vi "can test2.vi"() -> ()   [LabVIEW 2015]
uses:
  <vilib>/myRIO/Common/Instrument Driver Framework/myRIO v1.0/DIO/typedefs/DIO Channels Enum.ctl
  <vilib>/myRIO/Common/Instrument Driver Framework/myRIO v1.0/DIO/typedefs/DIO Channels List.ctl
  <vilib>/myRIO/Common/Instrument Driver Framework/Utilities/typedefs/Generic FPGA Reference.ctl
  <vilib>/myRIO/Common/Instrument Driver Framework/Utilities/typedefs/myRIO v1.0 Reference.ctl
  <vilib>/myRIO/Common/Instrument Driver Framework/Utilities/typedefs/Hardware Version Enum.ctl
  <vilib>/myRIO/Common/Instrument Driver Framework/Utilities/typedefs/myRIO Generic Hardware Reference.ctl
  <vilib>/myRIO/Instrument Drivers/Onboard IO/DIO/typedefs/DIO Reference.ctl
  <vilib>/myRIO/Instrument Drivers/Onboard IO/DIO/DIO.lvlib
  <vilib>/myRIO/Instrument Drivers/Onboard IO/DIO/vis/myRIO DIO Open.xnode
  <vilib>/myRIO/Common/Instrument Driver Framework/myRIO v1.0/DIO/vis/myRIO v1.1 Open DIO.vi
  <vilib>/userdefined/High Color/nirio_resource_hc.ctl
  <vilib>/myRIO/Instrument Drivers/Onboard IO/PWM/PWM.lvlib
  <vilib>/myRIO/Instrument Drivers/Onboard IO/AO/AO.lvlib
  rio_Global.vi
  <vilib>/Analysis/Matrix/NI_Matrix.lvlib
  <vilib>/Analysis/Matrix/Numeric/Conversions/Array To Matrix - RA2.vi
  <vilib>/Analysis/Matrix/Numeric/Multiply/Multiply - RM,RM.vi
  <vilib>/Analysis/Matrix/Numeric/Add/Add - RM,RM.vi
  <vilib>/Analysis/NI_AALBase.lvlib
  <vilib>/Analysis/baseanly.llb/Real Inverse Matrix.vi
  <vilib>/Analysis/Matrix/Numeric/Subtract/Subtract - RM,RM.vi
  <vilib>/Analysis/Matrix/Numeric/Conversions/Array To Matrix - RA.vi
  <vilib>/Analysis/Matrix/Numeric/Conversions/Matrix To Array - RM.vi
  <vilib>/Analysis/Matrix/Numeric/Multiply/Multiply - R,RM.vi
panel:
  out "Ring":u16(ring) items=["P", "R", "N", "D"]
  out "current gear":string(combo)
  in  "gear input":string(combo)
  in  "upper limit":dbl=1.0 format="%#_13g"
  out "XY Graph":cluster{"Y":dbl[], "Y":dbl[]}[](graph)=[{"Y"=[1.82421875, 1.8301353427767753, 1.835194070339203, 1.8394013252854347, 1.8427635002136231, 1.84528698772192, 1.8469781804084777, 1.8478434708714486, 1.8478892517089844, 1.8471219155192375, 1.84554785490036, 1.8431734624505043, 1.8400051307678222, 1.8360492524504661, 1.8313122200965881, 1.8258004263043404, 1.819520263671875, 1.8124781247973443, 1.8046804022789003, 1.796133488714695, 1.7868437767028809, 1.77681765884161, 1.7660615277290344, 1.7545817759633064, 1.742384796142578, 1.7294769808650017, 1.7158647227287291, 1.701554414331913, 1.686552448272705, 1.6708652171492577, 1.654499113559723, 1.637460530102253, 1.619755859375, 1.6013914939761162, 1.5823738265037537, 1.5627092495560646, 1.5424041557312012, 1.5214649376273155, 1.4998979878425598, 1.4777096989750862, 1.4549064636230469, 1.431494674384594, 1.4074807238578795, 1.3828710046410562, 1.3576719093322753, 1.3318898305296898, 1.3055311608314515, 1.2786022928357124, 1.251109619140625, 1.2230595323443412], "Y"=[0.0, 0.5, 1.0, 1.5, 2.0, 2.5, 3.0, 3.5, 4.0, 4.5, 5.0, 5.5, 6.0, 6.5, 7.0, 7.5, 8.0, 8.5, 9.0, 9.5, 10.0, 10.5, 11.0, 11.5, 12.0, 12.5, 13.0, 13.5, 14.0, 14.5, 15.0, 15.5, 16.0, 16.5, 17.0, 17.5, 18.0, 18.5, 19.0, 19.5, 20.0, 20.5, 21.0, 21.5, 22.0, 22.5, 23.0, 23.5, 24.0, 24.5]}, {"Y"=[-1.22265625, -1.2167396572232247, -1.211680929660797, -1.2074736747145653, -1.2041114997863769, -1.20158801227808, -1.1998968195915223, -1.1990315291285514, -1.1989857482910156, -1.1997530844807625, -1.20132714509964, -1.2037015375494957, -1.2068698692321778, -1.2108257475495339, -1.2155627799034119, -1.2210745736956596, -1.227354736328125, -1.2343968752026557, -1.2421945977210997, -1.250741511285305, -1.2600312232971191, -1.27005734115839, -1.2808134722709656, -1.2922932240366936, -1.304490203857422, -1.3173980191349983, -1.3310102772712709, -1.345320585668087, -1.360322551727295, -1.3760097828507423, -1.392375886440277, -1.409414469897747, -1.427119140625, -1.4454835060238838, -1.4645011734962463, -1.4841657504439354, -1.5044708442687988, -1.5254100623726845, -1.5469770121574402, -1.5691653010249138, -1.5919685363769531, -1.615380325615406, -1.6393942761421205, -1.6640039953589438, -1.6892030906677247, -1.7149851694703102, -1.7413438391685485, -1.7682727071642876, -1.795765380859375, -1.8238154676556588, -1.8524165749549866, -1.8815623101592065, -1.911246280670166, -1.9414620938897134, -1.972203357219696, -2.003463678061962, -2.0352366638183597, -2.0675159218907355, -2.1002950596809384, -2.1335676845908162, -2.167327404022217, -2.2015678253769875, -2.2362825560569766, -2.2714652034640315, -2.307109375, -2.3432086780667305, -2.3797567200660703, -2.4167471083998677, -2.4541734504699706, -2.4920293536782263, -2.530308425426483, -2.5690042731165885, -2.6081105041503907, -2.647620725929737, -2.687528545856476, -2.7278275713324547, -2.7685114097595216, -2.809573668539524, -2.8510079550743104, -2.892807876765728, -2.934967041015625, -2.977479055225849, -3.020337526798248, -3.0635360631346704, -3.107068271636963, -3.150927759706974, -3.1951081347465515, -3.2396030041575434, -3.284405975341797, -3.3295106557011604, -3.3749106526374817, -3.4205995735526087, -3.466571025848389, -3.51281861692667, -3.5593359541893004], "Y"=[0.0, 0.5, 1.0, 1.5, 2.0, 2.5, 3.0, 3.5, 4.0, 4.5, 5.0, 5.5, 6.0, 6.5, 7.0, 7.5, 8.0, 8.5, 9.0, 9.5, 10.0, 10.5, 11.0, 11.5, 12.0, 12.5, 13.0, 13.5, 14.0, 14.5, 15.0, 15.5, 16.0, 16.5, 17.0, 17.5, 18.0, 18.5, 19.0, 19.5, 20.0, 20.5, 21.0, 21.5, 22.0, 22.5, 23.0, 23.5, 24.0, 24.5, 25.0, 25.5, 26.0, 26.5, 27.0, 27.5, 28.0, 28.5, 29.0, 29.5, 30.0, 30.5, 31.0, 31.5, 32.0, 32.5, 33.0, 33.5, 34.0, 34.5, 35.0, 35.5, 36.0, 36.5, 37.0, 37.5, 38.0, 38.5, 39.0, 39.5, 40.0, 40.5, 41.0, 41.5, 42.0, 42.5, 43.0, 43.5, 44.0, 44.5, 45.0, 45.5, 46.0, 46.5, 47.0]}, {"Y"=[-0.94, 0.94, 0.94, -0.94, -0.94], "Y"=[-3.2, -3.2, 1.5, 1.5, -3.2]}, {"Y"=[1.984375, 1.978057861328125, 1.9718017578125, 1.965606689453125, 1.95947265625], "Y"=[0.0, 0.5, 1.0, 1.5, 2.0]}, {"Y"=[-5.28125, -5.267578125, -5.25390625, -5.240234375, -5.2265625], "Y"=[0.0, 0.5, 1.0, 1.5, 2.0]}]
  out "Heading":dbl
  out "H_GPS":dbl
  out "pos":dbl[](array[numeric])
  in  "GPS init":bool=TRUE
  out "pos_gps":dbl[](array[numeric]) format="%#_19f"
  out "dt":dbl
  out "Pos_time 10":i32
  out "ecef ref":dbl[](array[numeric])
  out "map":i32=2
  out "vgain":dbl=1.0
  out "vcount":u64=1
  out "hbias":dbl
  out "hcount":u64=1
  out "get heading":bool
  out "get position":bool
  out "heading error":dbl
  out "h_gps":dbl
  out "rt":dbl
  out "pos error":dbl
  out "POS init":bool
  out "Numeric":dbl
  out "cmd steer":dbl=25.77230806 format="%#_12g"
  in  "lane center":dbl=0.05 format="%#_13g"
  in  "Kf":dbl=0.18 format="%#_13g"
  out "Waveform Chart":dynamicdata(graph)
  out "mdps torque volt":dbl
  out "recomammed Speed [km/h]":dbl
  out "lane both":bool
  in  "gain(<1)":dbl=1.0 format="%#_13g"
  in  "rate limit":dbl=0.006 format="%#_13g"
  in  "deadzone":dbl
  in  "visco":dbl
  in  "Kp":dbl=1.2 format="%#_13g"
  out "VS_CAN":dbl
  out "car":refnum<k5>
  in  "forgetting":dbl format="%#_13g"
  out "mdps str_ang":dbl
  out "eye":refnum<k5>
  out "APV":dbl
  out "PWM GAS":dbl=1000.0 min=1000.0 max=2000.0 step=1.0
  out "Auto":bool
  in  "Manual Steering torque":dbl(slide) min=-0.3 max=0.3 step=0.01 scale=-0.3..0.3
  in  "Steering torque input":bool
  out "T init":i32
  out "T out":i32
  in  "manual speed":dbl
  in  "Velocity input":bool
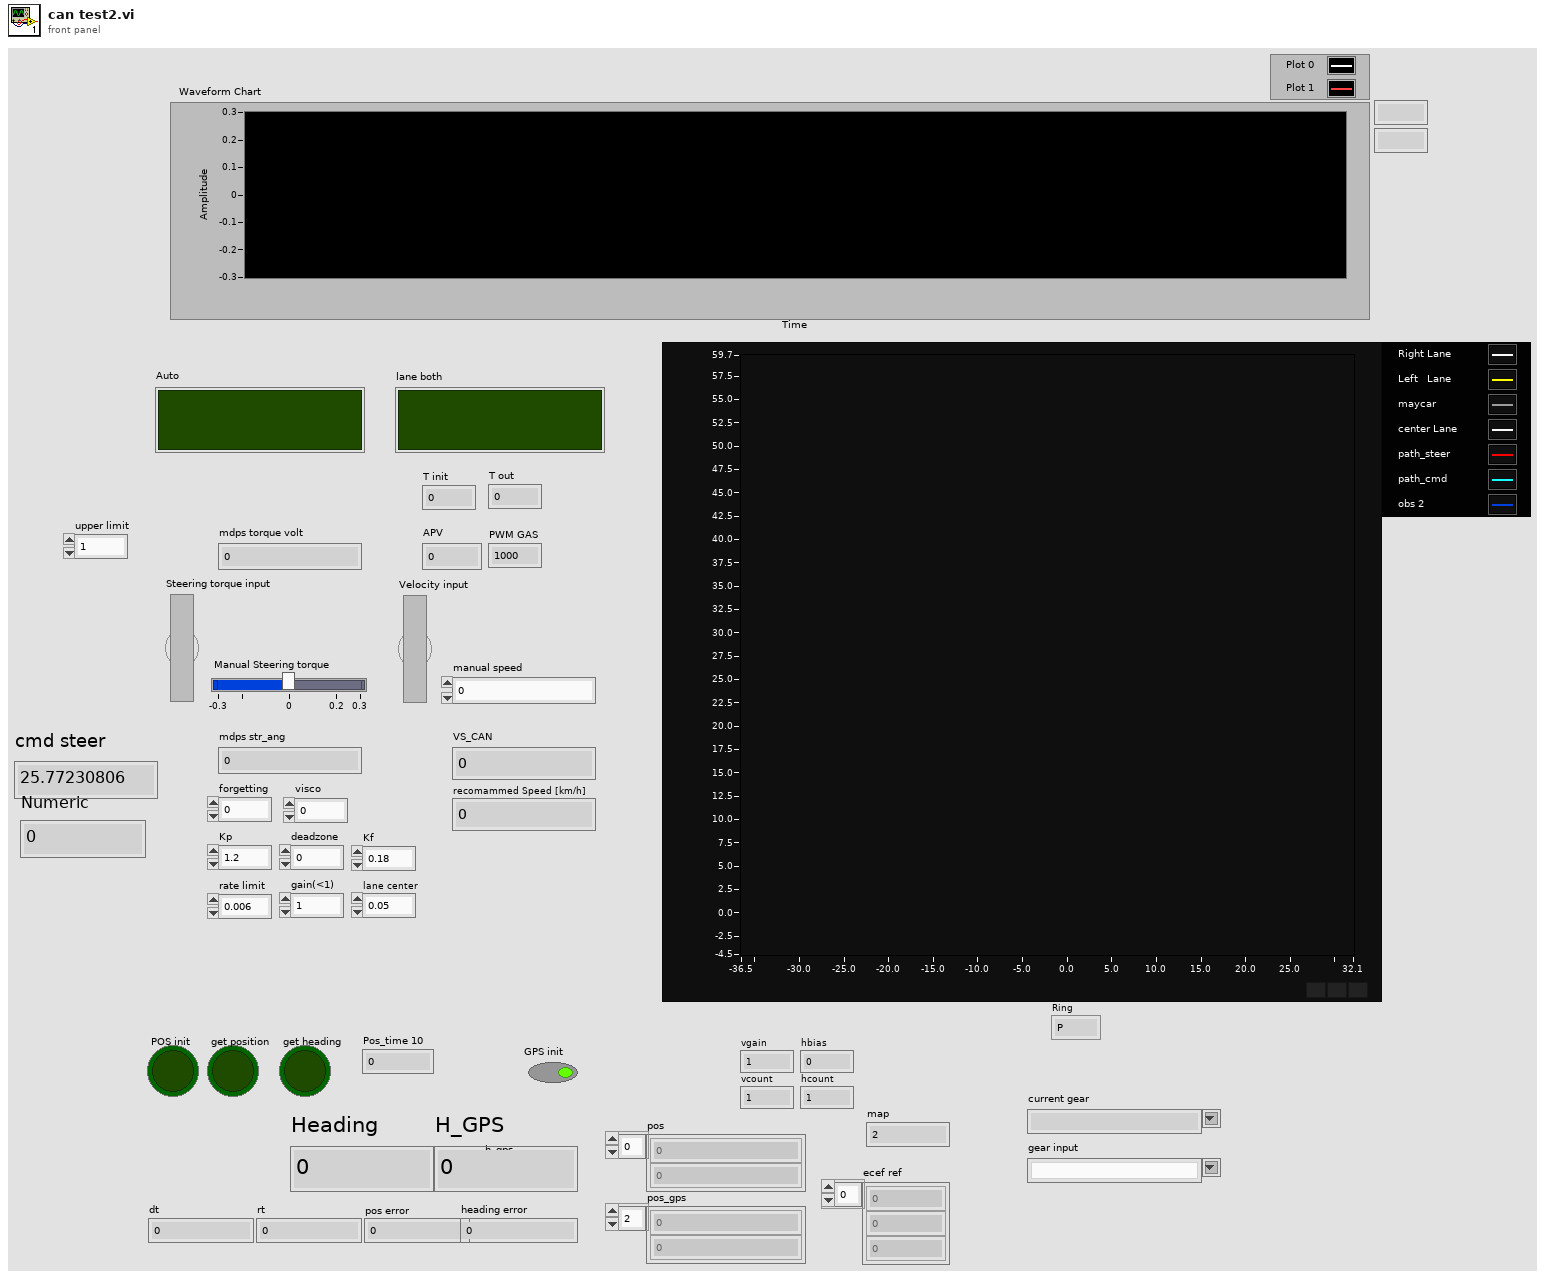
[diagram p1: front panel]
types:
  T1 = enum16{"Standard", "Buffered", "CRLF", "Immediate"}
  T2 = cluster{"identifier":u32, "timestamp":timestamp, "payload":u8[]}
  T3 = typedef "nirio_resource_hc.ctl" = tag
  T4 = typedef "Hardware Version Enum.ctl" = enum16{"Unknown", "myRIO-1900", "myRIO-1950", "roboRIO"}
  T5 = cluster{"connection ID":refnum<k16>, "net address":u32, "port":u16}
  T6 = cluster{"hash":i64, "sys time":i64, "mobileye time":u32, "ID":u32, "data":u8[]}
  T7 = cluster{"hash":i64, "sys time":i64, "car time":u32, "ID":u32, "data":u8[]}
  T8 = typedef "AO.lvlib/AO Reference.ctl" = cluster{"myRIO Reference":T9, "AO Channel List":T12, "AO Scaling Constant List":T14}
  T9 = typedef "myRIO Generic Hardware Reference.ctl" = cluster{"myRIO Model":T4, "myRIO Hardware Reference":T10}
  T10 = typedef "myRIO v1.0 Reference.ctl" = cluster{"Generic FPGA Reference":T11, "Allow multiple opens":bool}
  T11 = typedef "Generic FPGA Reference.ctl" = refnum<k20>
  T12 = typedef "AO Channels List.ctl" = T13[]
  T13 = typedef "AO Channels Enum.ctl" = enum16{"Not Connected", "AudioOut/Left", "AudioOut/Right", "C/AO0", "C/AO1", "A/AO0", "A/AO1", "B/AO0", "B/AO1"}
  T14 = typedef "Analog Scaling Constants List.ctl" = T15[]
  T15 = typedef "Analog Scaling Constants.ctl" = cluster{"LSB Weight (Volts)":dbl, "Offset (Volts)":dbl, "Signed?":bool}
  T16 = typedef "PWM.lvlib/PWM Reference.ctl" = cluster{"myRIO Reference":T9, "PWM Channels Enum":T17, "PWM Configuration":T18}
  T17 = typedef "PWM Channels Enum.ctl" = enum16{"Not Connected", "C/PWM0", "C/PWM1", "A/PWM0", "A/PWM1", "A/PWM2", "B/PWM0", "B/PWM1", "B/PWM2", "PWM/PWM0", "PWM/PWM1", "PWM/PWM2", "PWM/PWM3", "PWM/PWM4", "PWM/PWM5", "PWM/PWM6", "PWM/PWM7", "PWM/PWM8", "PWM/PWM9"}
  T18 = typedef "PWM.lvlib/PWM Configuration.ctl" = cluster{"Frequency":dbl, "Duty Cycle":dbl}
  T19 = typedef "DIO.lvlib/DIO Reference.ctl" = cluster{"myRIO Reference":T9, "DIO Channels List":T20}
  T20 = typedef "DIO Channels List.ctl" = T21[]
  T21 = typedef "DIO Channels Enum.ctl" = enum16{"Not Connected", "C/DIO0", "C/DIO1", "C/DIO2", "C/DIO3", "C/DIO4", "C/DIO5", "C/DIO6", "C/DIO7", "A/DIO0", "A/DIO1", "A/DIO2", "A/DIO3", "A/DIO4", "A/DIO5", "A/DIO6", "A/DIO7", "A/DIO8", "A/DIO9", "A/DIO10", "A/DIO11", "A/DIO12", "A/DIO13", "A/DIO14", "A/DIO15", "B/DIO0", "B/DIO1", "B/DIO2", "B/DIO3", "B/DIO4", "B/DIO5", "B/DIO6", "B/DIO7", "B/DIO8", "B/DIO9", "B/DIO10", "B/DIO11", "B/DIO12", "B/DIO13", "B/DIO14", "B/DIO15", "LED0", "LED1", "LED2", "LED3", "Button0", "DIO/DIO0", "DIO/DIO1", "DIO/DIO2", "DIO/DIO3", "DIO/DIO4", "DIO/DIO5", "DIO/DIO6", "DIO/DIO7", "DIO/DIO8", "DIO/DIO9", "SPI/CS0", "SPI/CS1", "SPI/CS2", "SPI/CS3", "LED RADIO (Green)", "LED RADIO (Red)", "LED COMM (Green)", "LED COMM (Red)", "LED MODE (Green)", "LED MODE (Red)"}
  T22 = cluster{"hash":i64, "sys time":i64, "ref_vel":dbl, "ref_steer":dbl}
  T23 = cluster{"hash":i64, "sys time":i64, "time":dbl, "x":dbl, "y":dbl, "h":dbl, "numSV":i32, "postype":i32, "lag":i32, "hordev":dbl, "lat":dbl, "lon":dbl, "hgt":dbl, "map_idx":i32}
  T24 = cluster{"output[0]":dbl, "output[1]":dbl, "output[2]":dbl, "output[3]":dbl, "output[4]":dbl, "output[5]":dbl, "output[6]":dbl, "output[7]":dbl, "output[8]":dbl, "output[9]":dbl, "output[10]":dbl, "output[11]":dbl, "output[12]":dbl, "output[13]":dbl, "output[14]":dbl}
  T25 = cluster{"hash":i64, "sys time":i64, "time":dbl, "speed":dbl, "heading":dbl, "lat":dbl, "lon":dbl}
  T26 = cluster{"output[0]":dbl, "output[1]":dbl, "output[2]":dbl, "output[3]":dbl, "output[4]":dbl, "output[5]":dbl, "output[6]":dbl}
  T27 = typedef "NI_Matrix.lvlib/RealMatrix.ctl" = dbl[][]
  T28 = cluster{"hash":i64, "sys time":i64, "dt":dbl, "x":dbl, "y":dbl, "speed":dbl, "heading":dbl, "yaw_rate":dbl}
  T29 = cluster{"Real 2D Array[0]":dbl, "Real 2D Array[1]":dbl, "Real 2D Array[2]":dbl, "Real 2D Array[3]":dbl, "Real 2D Array[4]":dbl}
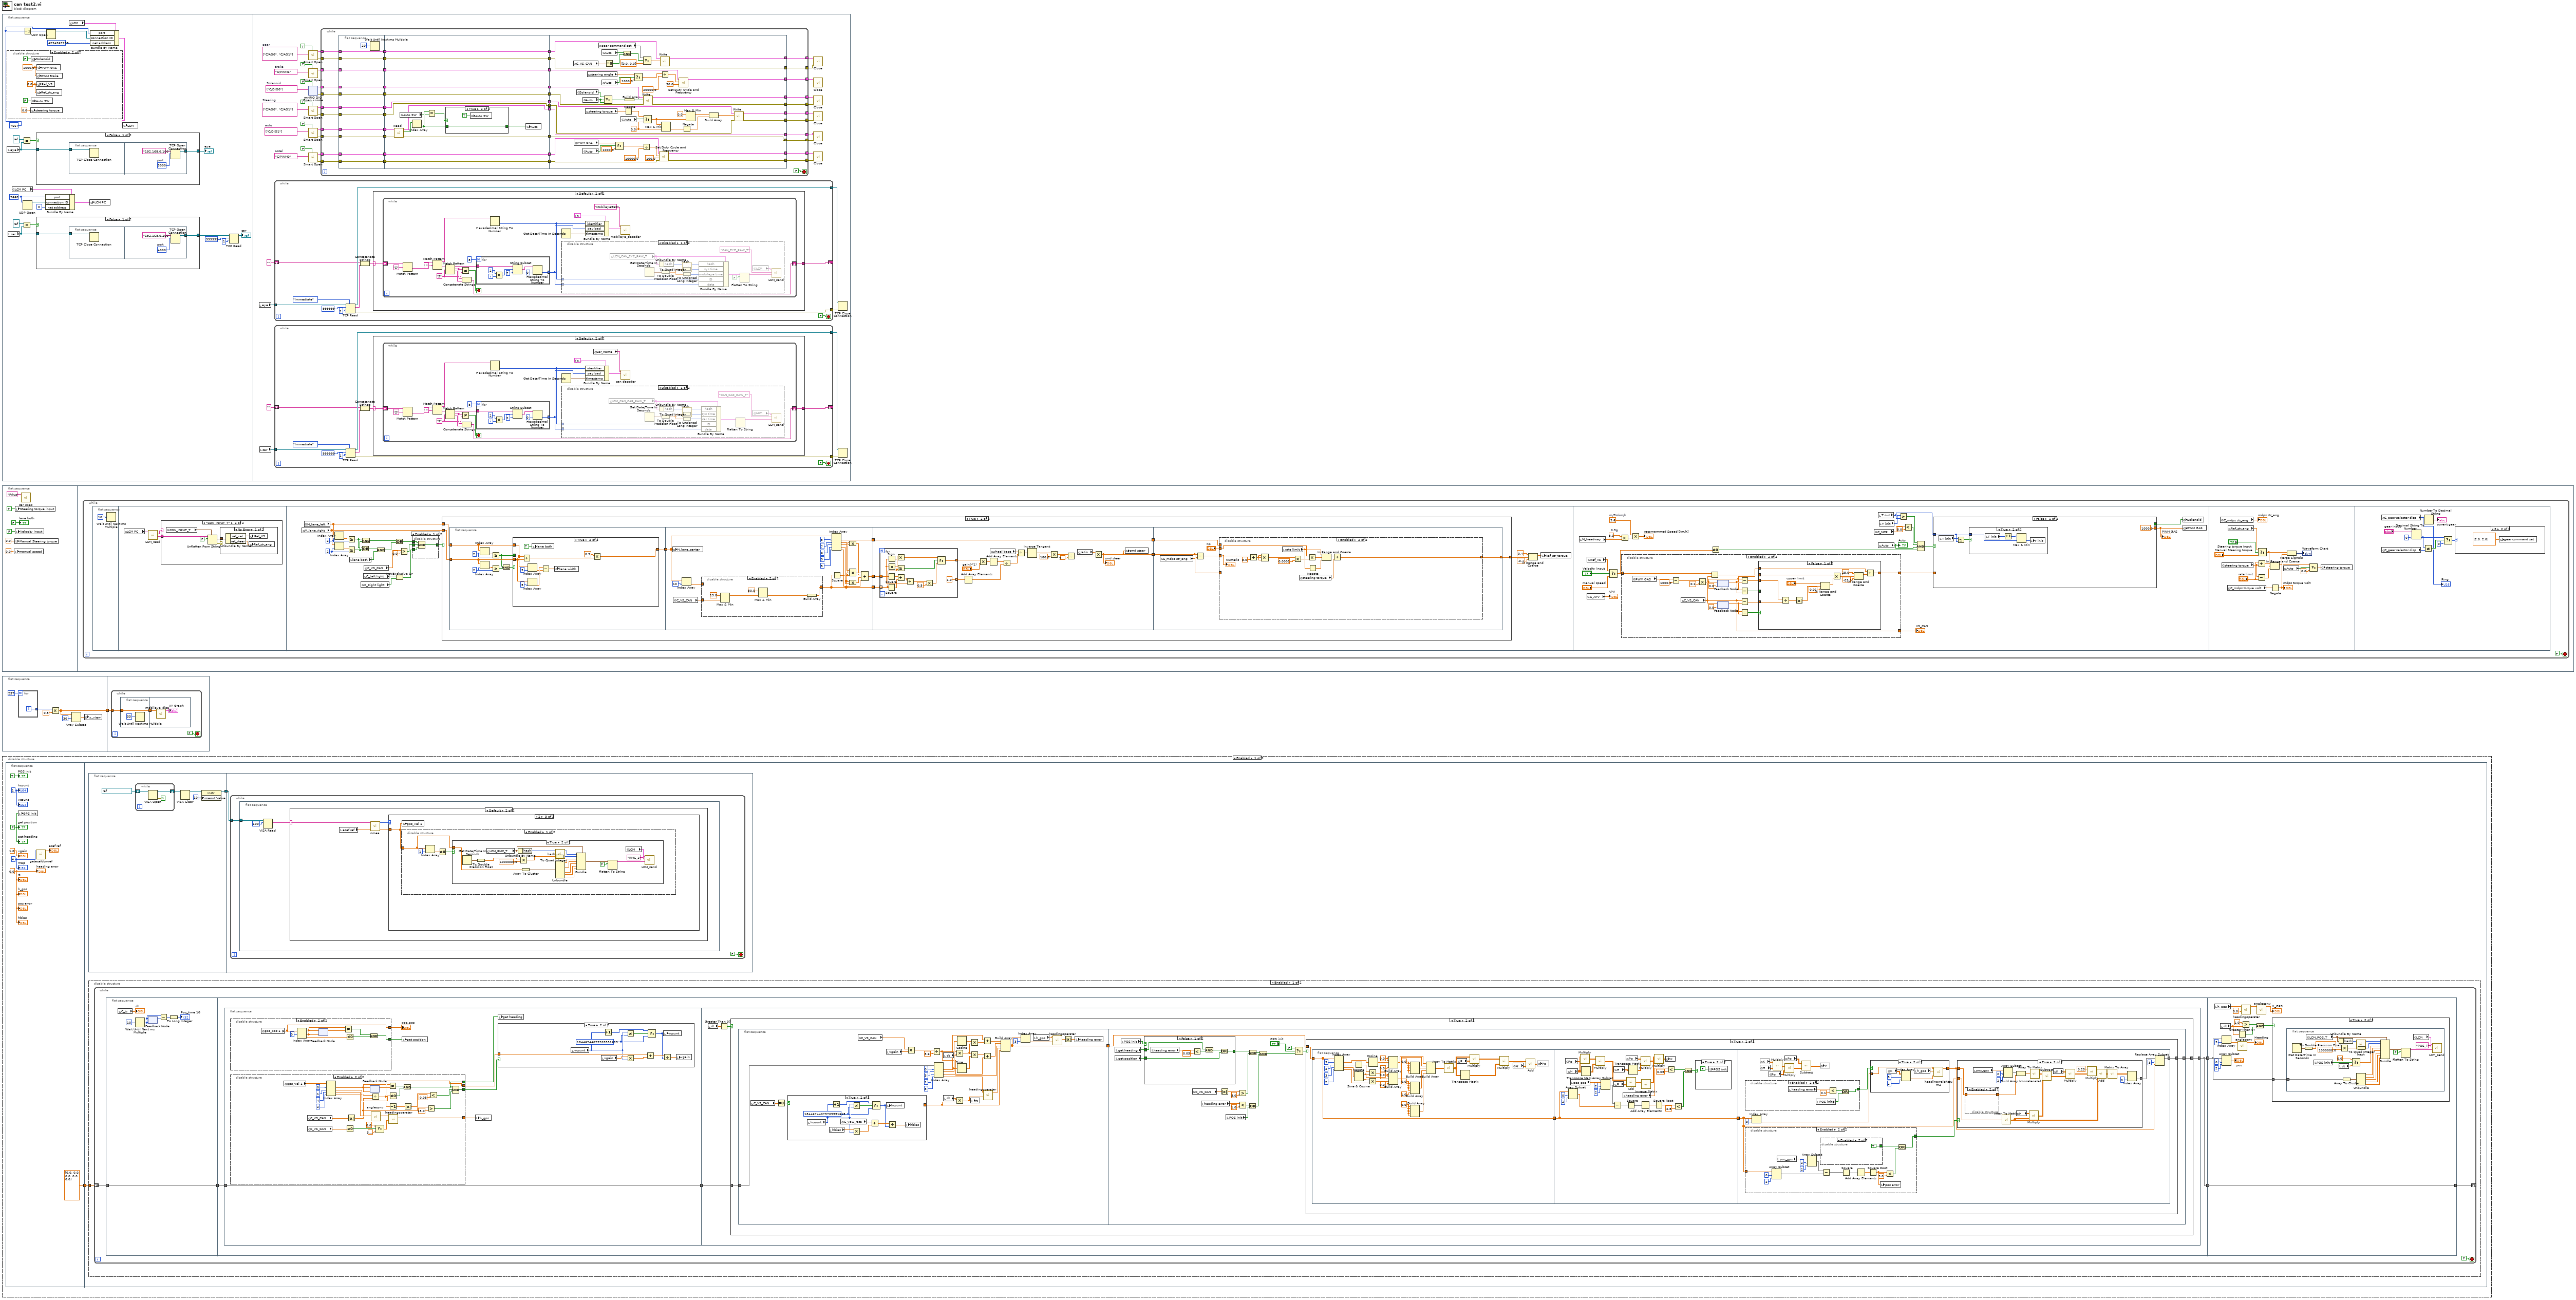
[diagram p0: block diagram]
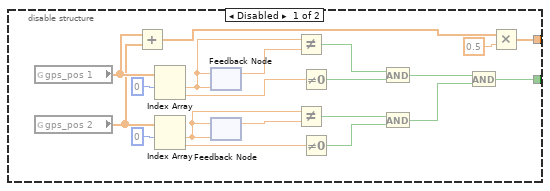
[diagram p2: hidden frame]
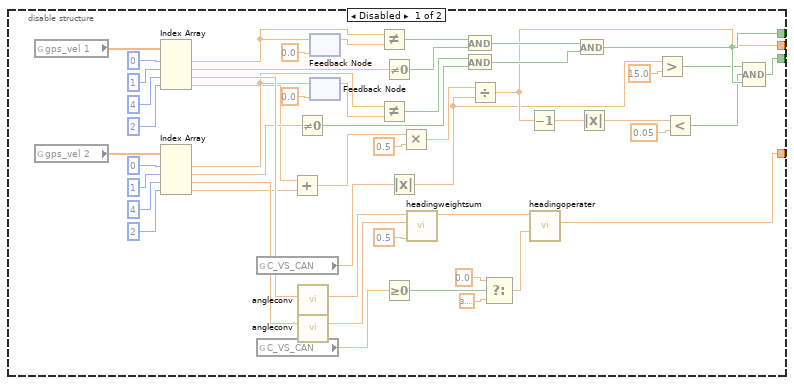
[diagram p3: hidden frame]
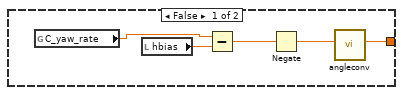
[diagram p6: hidden frame]
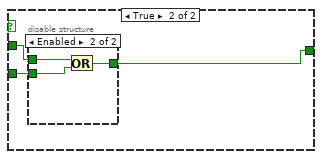
[diagram p7: hidden frame]
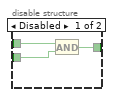
[diagram p8: hidden frame]
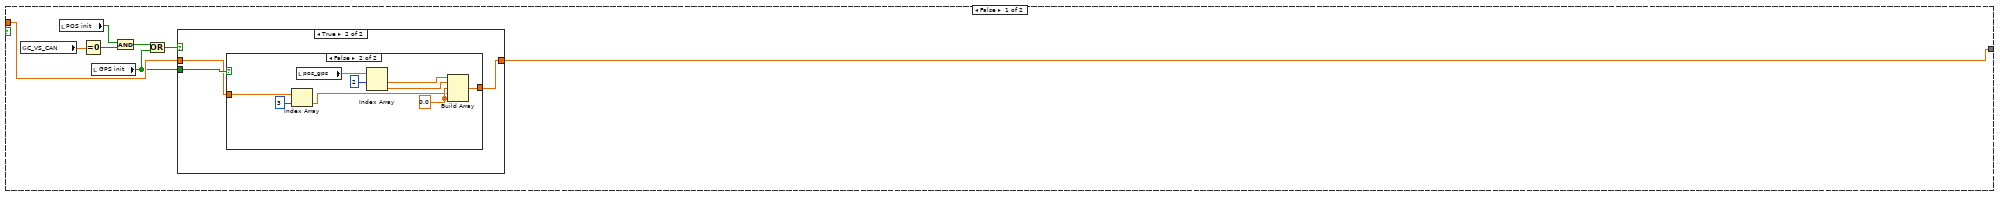
[diagram p9: hidden frame]
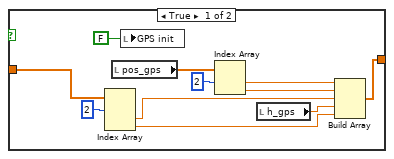
[diagram p11: hidden frame]
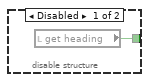
[diagram p13: hidden frame]
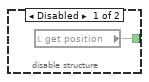
[diagram p14: hidden frame]
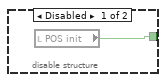
[diagram p15: hidden frame]
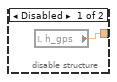
[diagram p17: hidden frame]
diagram:
  n1 = flat-sequence {
    frame #0 {
      w16 = u16 7668 ("port")
      w11 = u16 7667 ("port")
      n2 = disable-structure shown="Enabled" {
        frame Disabled {
        }
        frame Enabled {
          w24 = 0.0 ("Ref_str_ang")
          w25 = 1000.0 ("PWM GAS")
          n3 = global write "rio_Global.vi" "steering torque"(0.0 ("steering")) -> ()
          n4 = global write "rio_Global.vi" "Solenoid"(FALSE ("CAN A 1")) -> ()
          n5 = global write "rio_Global.vi" "Auto SW"(FALSE ("Auto SW")) -> ()
          n6 = global write "rio_Global.vi" "PWM Brake"(w25) -> ()
          n7 = global write "rio_Global.vi" "Ref_str_ang"(w24) -> ()
          n8 = global write "rio_Global.vi" "PWM GAS"(w25) -> ()
          n9 = global write "rio_Global.vi" "Ref_VS"(w24) -> ()
        }
      }
      n10 = local read "eye"() -> (w18:refnum<k5>)
      n11 = local read "car"() -> (w19:refnum<k5>)
      n12 = global read "rio_Global.vi" "LCM PC"() -> (w8:T5)
      n13 = Equal?(x=refnum<k5> refnum ("connection ID"), y=w18) -> (x = y?=w20:bool)
      n14 = Equal?(x=refnum<k5> refnum ("connection ID"), y=w19) -> (x = y?=w22:bool)
      n15 = Decrement(x=w11) -> (x-1=w10:u16)
      n16 = UDP Open(11:w16) -> (port=w14:refnum<k16>)  [unwired: 4 in, 2 out]
      n17 = case shown="False" w20 {
        tunnel: w18 -> [w30 _]
        tunnel: [w29 w35] -> w17
        frame False {
          n18 = flat-sequence {
            tunnel: w30 -> [w31]
            tunnel: [w32] -> w29
            frame #0 {
              n19 = TCP Close Connection(connection ID=w31) -> ()  [unwired: 2 in, 2 out]
            }
            frame #1 {
              w33 = u16 3000  # port
              n20 = TCP Open Connection(address="192.168.0.100", remote port or service name=w33) -> (connection ID=w32:refnum<k5>)  [unwired: 3 in, 1 out]
            }
          }
        }
        frame True {
          w36 = u16 3000  # port
          n21 = TCP Open Connection(address="192.168.0.100", remote port or service name=w36) -> (connection ID=w35:refnum<k5>)  [unwired: 3 in, 1 out]
        }
      }
      "eye" <- w17
      n22 = case shown="False" w22 {
        tunnel: w19 -> [w39 _]
        tunnel: [w38 w44] -> w3
        frame False {
          n23 = flat-sequence {
            tunnel: w39 -> [w40]
            tunnel: [w41] -> w38
            frame #0 {
              n24 = TCP Close Connection(connection ID=w40) -> ()  [unwired: 2 in, 2 out]
            }
            frame #1 {
              w42 = u16 4000  # port
              n25 = TCP Open Connection(address="192.168.0.200", remote port or service name=w42) -> (connection ID=w41:refnum<k5>)  [unwired: 3 in, 1 out]
            }
          }
        }
        frame True {
          w45 = u16 4000  # port
          n26 = TCP Open Connection(address="192.168.0.200", remote port or service name=w45) -> (connection ID=w44:refnum<k5>)  [unwired: 3 in, 1 out]
        }
      }
      n27 = Bundle By Name(cluster=w8, "port"=w16, "connection ID"=w14, "net address"=u32 0) -> (w9:T5)
      n28 = UDP Open(11:w10) -> (port=w13:refnum<k16>)  [unwired: 4 in, 2 out]
      n29 = global read "rio_Global.vi" "LCM"() -> (w7:T5)
      n30 = global write "rio_Global.vi" "LCM PC"(w9) -> ()
      n31 = Bundle By Name(cluster=w7, "port"=w11, "connection ID"=w13, "net address"=u32 4294967295) -> (w6:T5)
      n32 = global write "rio_Global.vi" "LCM"(w6) -> ()
      n33 = TCP Read(connection ID=w3, bytes to read=999999, 9:1 ("timeout ms (25000)")) -> (connection ID out=→"car":refnum<k5>)  [unwired: 2 in, 2 out]
    }
    frame #1 {
      w52 = tag[] ["C/AO0", "C/AO1"]  # gear
      w56 = tag "C/PWM1"  # Brake
      w70 = tag[] ["C/AO0", "C/AO1"]  # Steering
      w77 = tag[] ["C/DIO1"]  # auto
      w82 = tag "C/PWM0"  # Accel
      w87 = tag[] ["C/DIO0"]  # Solenoid
      n34 = local read "eye"() -> (w61:refnum<k5>)
      n35 = local read "car"() -> (w57:refnum<k5>)
      n36 = while {
        tunnel: w61 -> [w146]
        tunnel: [w148] -> w64
        tunnel: [w147] -> w63
        shift-right: [w142] -> _
        shift-left: "" -> [w145]
        stop <- FALSE stop-if-true
        n37 = TCP Read(connection ID=w146, bytes to read=999999, 7:T1."Immediate" ("mode (standard)"), 9:1 ("timeout ms (25000)")) -> (connection ID out=w148:refnum<k5>, data out=w144:string, error out=w147:errorcluster)  [unwired: 1 in]
        n38 = Concatenate Strings(w145, w144) -> (w143:string)
        n39 = case shown="Default" w143 {
          selector: w143 -> [_ w154]
          tunnel: [_ w153] -> w142
          frame "" {
          }
          frame Default {
            n40 = while {
              shift-right: [w161] -> w153
              shift-left: w154 -> [w173]
              stop <- w158 stop-if-true
              w159 = "S" ("regular expression")
              n41 = Match Pattern(string=w173, regular expression="S") -> (after substring=w171:string)  [unwired: 1 in, 3 out]
              n42 = Match Pattern(string=w171, regular expression=" ") -> (before substring=w169:string, after substring=w166:string)  [unwired: 1 in, 2 out]
              n43 = Match Pattern(string=w166, regular expression=w159) -> (before substring=w165:string, match substring=w160:string, after substring=w162:string)  [unwired: 1 in, 1 out]
              n44 = Not Equal?(x=w160, y=w159) -> (x != y?=w158:bool)
              n45 = Concatenate Strings(w160, w162) -> (w161:string)
              n46 = for {
                N: 8 -> [_]
                tunnel: w165 -> [w195]
                tunnel: [w191] -> w155 mode=indexing
                i -> [w190]
                n47 = Multiply(x=2, y=w190) -> (x*y=w193:i32)
                n48 = String Subset(string=w195, offset (0)=w193, length (rest)=2 ("length (rest)")) -> (substring=w188:string)
                n49 = Hexadecimal String To Number(string=w188, default (0uL)=u8 0) -> (number=w191:u8)  [unwired: 1 in, 1 out]
              }
              n50 = Hexadecimal String To Number(string=w169) -> (number=w156:u32)  [unwired: 2 in, 1 out]
              n51 = Get Date/Time In Seconds() -> (seconds since 1Jan1904=w164:timestamp)
              n52 = disable-structure shown="Disabled" {
                disable-tunnel: w156 -> [w175 _]
                disable-tunnel: w155 -> [w174 _]
                frame Disabled {
                  n53 = global read "rio_Global.vi" "LCM_CAN_EYE_RAW_T"() -> (w182:T6)
                  n54 = Get Date/Time In Seconds() -> (seconds since 1Jan1904=w179:timestamp)
                  n55 = Unbundle By Name(w182) -> ("hash"=w181:i64)
                  n56 = To Double Precision Float(number=w179) -> (double precision float=w177:dbl)
                  n57 = To Quad Integer(1:w177) -> (0:w178:i64)
                  n58 = To Unsigned Long Integer(number=w177) -> (unsigned 32bit integer=w176:u32)
                  n59 = call "hash.vi"("input"=w181) -> ("output"=w183:i64)  [unwired: 10 in]
                  n60 = Bundle By Name(cluster=w182, "hash"=w183, "sys time"=w178, "mobileye time"=w176, "ID"=w175, "data"=w174) -> (w185:T6)
                  n61 = Flatten To String(anything=w185, prepend array or string size? (T)=FALSE) -> (data string=w187:string)  [unwired: 2 in, 2 out]
                  n62 = global read "rio_Global.vi" "LCM"() -> (w186:T5)
                  n63 = call "LCM_send.vi"("DATA"=w187, "ID"="CAN_EYE_RAW_T", "LCM"=w186) -> ()  [unwired: 6 in, 3 out]
                }
                frame Enabled {
                }
              }
              n64 = Bundle By Name(cluster=T2 {"identifier"=0, "timestamp"=timestamp(0 s since 1904-01-01), "payload"=[]} ("can cluster"), "identifier"=w156, "payload"=w155, "timestamp"=w164) -> (w163:T2)
              n65 = call "mobileye_decoder.vi"("can cluster"=w163, "name"="Mobileye560") -> ()  [unwired: 10 in]
            }
          }
        }
      }
      n66 = while {
        tunnel: w57 -> [w93]
        tunnel: [w95] -> w58
        tunnel: [w94] -> w59
        shift-right: [w89] -> _
        shift-left: "" -> [w92]
        stop <- FALSE stop-if-true
        n67 = TCP Read(connection ID=w93, bytes to read=999999, 7:T1."Immediate" ("mode (standard)"), 9:1 ("timeout ms (25000)")) -> (connection ID out=w95:refnum<k5>, data out=w91:string, error out=w94:errorcluster)  [unwired: 1 in]
        n68 = Concatenate Strings(w92, w91) -> (w90:string)
        n69 = case shown="Default" w90 {
          selector: w90 -> [_ w101]
          tunnel: [_ w100] -> w89
          frame "" {
          }
          frame Default {
            n70 = while {
              shift-right: [w110] -> w100
              shift-left: w101 -> [w120]
              stop <- w106 stop-if-true
              w107 = "S" ("regular expression")
              n71 = Match Pattern(string=w120, regular expression="S") -> (after substring=w118:string)  [unwired: 1 in, 3 out]
              n72 = Match Pattern(string=w118, regular expression=" ") -> (before substring=w116:string, after substring=w114:string)  [unwired: 1 in, 2 out]
              n73 = Match Pattern(string=w114, regular expression=w107) -> (before substring=w113:string, match substring=w108:string, after substring=w111:string)  [unwired: 1 in, 1 out]
              n74 = Not Equal?(x=w108, y=w107) -> (x != y?=w106:bool)
              n75 = Concatenate Strings(w108, w111) -> (w110:string)
              n76 = for {
                N: 8 -> [_]
                tunnel: w113 -> [w141]
                tunnel: [w137] -> w103 mode=indexing
                i -> [w136]
                n77 = Multiply(x=2, y=w136) -> (x*y=w139:i32)
                n78 = String Subset(string=w141, offset (0)=w139, length (rest)=2 ("length (rest)")) -> (substring=w134:string)
                n79 = Hexadecimal String To Number(string=w134, default (0uL)=u8 0) -> (number=w137:u8)  [unwired: 1 in, 1 out]
              }
              n80 = Hexadecimal String To Number(string=w116) -> (number=w104:u32)  [unwired: 2 in, 1 out]
              n81 = Get Date/Time In Seconds() -> (seconds since 1Jan1904=w112:timestamp)
              n82 = disable-structure shown="Disabled" {
                disable-tunnel: w104 -> [w126 _]
                disable-tunnel: w103 -> [w125 _]
                frame Disabled {
                  n83 = global read "rio_Global.vi" "LCM_CAN_CAR_RAW_T"() -> (w131:T7)
                  n84 = Get Date/Time In Seconds() -> (seconds since 1Jan1904=w133:timestamp)
                  n85 = Unbundle By Name(w131) -> ("hash"=w132:i64)
                  n86 = To Double Precision Float(number=w133) -> (double precision float=w124:dbl)
                  n87 = To Quad Integer(1:w124) -> (0:w128:i64)
                  n88 = To Unsigned Long Integer(number=w124) -> (unsigned 32bit integer=w127:u32)
                  n89 = call "hash.vi"("input"=w132) -> ("output"=w130:i64)  [unwired: 10 in]
                  n90 = Bundle By Name(cluster=w131, "hash"=w130, "sys time"=w128, "car time"=w127, "ID"=w126, "data"=w125) -> (w129:T7)
                  n91 = Flatten To String(anything=w129) -> (data string=w121:string)  [unwired: 3 in, 2 out]
                  n92 = global read "rio_Global.vi" "LCM"() -> (w122:T5)
                  n93 = call "LCM_send.vi"("DATA"=w121, "ID"="CAN_CAR_RAW_T", "LCM"=w122) -> ()  [unwired: 6 in, 3 out]
                }
                frame Enabled {
                }
              }
              n94 = Bundle By Name(cluster=T2 {"identifier"=0, "timestamp"=timestamp(0 s since 1904-01-01), "payload"=[]} ("can cluster"), "identifier"=w104, "payload"=w103, "timestamp"=w112) -> (w109:T2)
              n95 = global read "rio_Global.vi" "Car_name"() -> (w102:string)
              n96 = call "can decoder.vi"("can cluster"=w109, "name"=w102) -> ()  [unwired: 10 in]
            }
          }
        }
      }
      n97 = call <vilib>:"Smart Open.vi"("Allow multiple opens?"=TRUE, "Channel Names"=w52) -> ("error out"=w49:errorcluster, "AO Ref Out"=w50:T8)  [unwired: 8 in]
      n98 = call <vilib>:"Smart Open.vi"("Allow multiple opens?"=FALSE, "Channel Name"=w56) -> ("PWM Ref Out"=w54:T16)  [unwired: 8 in, 1 out]
      n99 = xnode "myRIO DIO Open.xnode"("Allow multiple opens?"=FALSE, "Channel Names"=w87) -> ("error out"=w85:errorcluster, "DIO Ref Out"=w86:T19)  [unwired: 1 in]
      n100 = call <vilib>:"Smart Open.vi"("Allow multiple opens?"=TRUE, "Channel Names"=w70) -> ("error out"=w68:errorcluster, "AO Ref Out"=w69:T8)  [unwired: 8 in]
      n101 = call <vilib>:"Smart Open.vi"("Allow multiple opens?"=FALSE, "Channel Names"=w77) -> ("error out"=w75:errorcluster, "DIO Ref Out"=w76:T19)  [unwired: 8 in]
      n102 = call <vilib>:"Smart Open.vi"("Allow multiple opens?"=FALSE, "Channel Name"=w82) -> ("error out"=w80:errorcluster, "PWM Ref Out"=w81:T16)  [unwired: 8 in]
      n103 = while {
        tunnel: w86 -> [w255]
        tunnel: [w256] -> w84
        tunnel: w85 -> [w254]
        tunnel: [w250] -> w83
        tunnel: w76 -> [w248]
        tunnel: [w246] -> w74
        tunnel: w75 -> [w247]
        tunnel: [w245] -> w73
        tunnel: w69 -> [w244]
        tunnel: [w242] -> w67
        tunnel: w68 -> [w243]
        tunnel: [w241] -> w66
        tunnel: w81 -> [w252]
        tunnel: [w253] -> w79
        tunnel: w80 -> [w251]
        tunnel: [w249] -> w78
        tunnel: w54 -> [w221]
        tunnel: [w220] -> w53
        tunnel: w50 -> [w217]
        tunnel: [w216] -> w48
        tunnel: [w215] -> w47
        tunnel: w49 -> [w212]
        stop <- FALSE ("Auto") stop-if-true
        n104 = flat-sequence {
          tunnel: w243 -> [w261]
          tunnel: w244 -> [w262]
          tunnel: w247 -> [w263]
          tunnel: w248 -> [w264]
          tunnel: w251 -> [w265]
          tunnel: w252 -> [w266]
          tunnel: w254 -> [w267]
          tunnel: w255 -> [w268]
          tunnel: [w268] -> w240
          tunnel: [w267] -> w238
          tunnel: [w266] -> w236
          tunnel: [w265] -> w234
          tunnel: [w264] -> w232
          tunnel: [w263] -> w230
          tunnel: [w262] -> w228
          tunnel: [w261] -> w226
          tunnel: [w259] -> w222
          tunnel: w221 -> [w259]
          tunnel: [w258] -> w218
          tunnel: w217 -> [w258]
          tunnel: [w257] -> w213
          tunnel: w212 -> [w257]
          tunnel: w240 -> [w286]
          tunnel: [w286] -> w239
          tunnel: w238 -> [w285]
          tunnel: [w285] -> w237
          tunnel: w236 -> [w284]
          tunnel: [w284] -> w235
          tunnel: w234 -> [w283]
          tunnel: [w283] -> w233
          tunnel: w232 -> [w279]
          tunnel: [w277] -> w231
          tunnel: w230 -> [w278]
          tunnel: [w276] -> w229
          tunnel: w228 -> [w282]
          tunnel: [w282] -> w227
          tunnel: w226 -> [w281]
          tunnel: [w281] -> w225
          tunnel: [w271] -> w223
          tunnel: w222 -> [w271]
          tunnel: [w270] -> w219
          tunnel: w218 -> [w270]
          tunnel: [w269] -> w214
          tunnel: w213 -> [w269]
          tunnel: [w342] -> w256
          tunnel: [w339] -> w253
          tunnel: [w336] -> w250
          tunnel: [w335] -> w249
          tunnel: [w321] -> w246
          tunnel: [w320] -> w245
          tunnel: [w331] -> w242
          tunnel: [w330] -> w241
          tunnel: w239 -> [w341]
          tunnel: w237 -> [w340]
          tunnel: w235 -> [w338]
          tunnel: w233 -> [w337]
          tunnel: w231 -> [w321]
          tunnel: w229 -> [w320]
          tunnel: w227 -> [w333]
          tunnel: w225 -> [w332]
          tunnel: w223 -> [w306]
          tunnel: [w305] -> w220
          tunnel: w219 -> [w298]
          tunnel: [w297] -> w216
          tunnel: [w296] -> w215
          tunnel: w214 -> [w296]
          frame #0 {
            n105 = Wait Until Next ms Multiple(millisecond multiple=u32 20) -> ()  [unwired: 1 out]
          }
          frame #1 {
            n106 = call <vilib>:"Read.vi"("error in (no error)"=w278, "DIO Ref In"=w279) -> ("error out"=w276:errorcluster, "Values"=w280:bool[], "DIO Ref Out"=w277:T19)  [unwired: 7 in]
            n107 = global read "rio_Global.vi" "Auto SW"() -> (w273:bool)
            n108 = Index Array(array=w280) -> (element=w274:bool)  [unwired: 1 in]
            n109 = Equal?(x=w274, y=w273) -> (x = y?=w275:bool)
            n110 = case shown="True" w275 {
              tunnel: w274 -> [_ w288]
              tunnel: [_ w288] -> w272
              frame False {
              }
              frame True {
                n111 = global write "rio_Global.vi" "Auto SW"(TRUE ("Auto SW")) -> ()
              }
            }
            n112 = global write "rio_Global.vi" "Auto"(w272) -> ()
          }
          frame #2 {
            w318 = 0.0 ("y")
            n113 = global read "rio_Global.vi" "C_VS_CAN"() -> (w292:dbl)
            n114 = global read "rio_Global.vi" "PWM GAS"() -> (w308:dbl)
            n115 = global read "rio_Global.vi" "Solenoid"() -> (w310:bool)
            n116 = global read "rio_Global.vi" "Auto"() -> (w311:bool)
            n117 = global read "rio_Global.vi" "Auto"() -> (w312:bool)
            n118 = global read "rio_Global.vi" "steering torque"() -> (w309:dbl)
            n119 = global read "rio_Global.vi" "steering angle"() -> (w302:dbl)
            n120 = global read "rio_Global.vi" "gear command set"() -> (w295)
            n121 = global read "rio_Global.vi" "Auto"() -> (w290:bool)
            n122 = global read "rio_Global.vi" "Auto"() -> (w300:bool)
            n123 = Select(t=w310, s=w311, f=w311) -> (s? t:f=w314:bool)
            n124 = Equal To 0?(x=w292) -> (x = 0?=w291:bool)
            n125 = Select(t=w308, s=w312, f=1000.0) -> (s? t:f=w317:dbl)
            n126 = global read "rio_Global.vi" "Auto"() -> (w313:bool)
            n127 = And(x=w290, y=w291) -> (x .and. y?=w289:bool)
            n128 = Negate(x=w309) -> (-x=w315:dbl)
            n129 = Build Array(w314) -> (w325:bool[])
            n130 = Select(t=w302, s=w300, f=1000.0) -> (s? t:f=w301:dbl)
            n131 = Divide(x=w317, y=10000.0) -> (x/y=w322:dbl)
            n132 = Select(t=w295, s=w289, f=dbl[] [0.0, 0.0]) -> (s? t:f=w294:dbl[])
            n133 = Select(t=w315, s=w313, f=w318) -> (s? t:f=w319:dbl)
            n134 = call <vilib>:"Write.vi"("error in (no error)"=w340, "Values"=w325, "DIO Ref In"=w341) -> ("error out"=w336:errorcluster, "DIO Ref Out"=w342:T19)  [unwired: 6 in]
            n135 = call <vilib>:"Set Duty Cycle and Frequency.vi"("error in (no error)"=w337, "Frequency [Hz]"=100.0, "Duty Cycle"=w322, "PWM Ref In"=w338) -> ("error out"=w335:errorcluster, "PWM Ref Out"=w339:T16)  [unwired: 5 in]
            n136 = call <vilib>:"Write.vi"("Values"=w294, "AO Ref In"=w298) -> ("AO Ref Out"=w297:T8)  [unwired: 7 in, 1 out]
            n137 = Divide(x=w301, y=20000.0) -> (x/y=w304:dbl)
            n138 = Max & Min(x=w319, y=w318) -> (min(x,y)=w327:dbl)  [unwired: 1 out]
            n139 = call <vilib>:"Set Duty Cycle and Frequency.vi"("Frequency [Hz]"=50.0, "Duty Cycle"=w304, "PWM Ref In"=w306) -> ("PWM Ref Out"=w305:T16)  [unwired: 6 in, 1 out]
            n140 = Negate(x=w327) -> (-x=w326:dbl)
            n141 = Max & Min(x=0.0, y=w319) -> (max(x,y)=w328:dbl)  [unwired: 1 out]
            n142 = Build Array(w328, w326) -> (w334:dbl[])
            n143 = call <vilib>:"Write.vi"("error in (no error)"=w332, "Values"=w334, "AO Ref In"=w333) -> ("error out"=w330:errorcluster, "AO Ref Out"=w331:T8)  [unwired: 6 in]
          }
        }
      }
      n144 = call <vilib>:"Close.vi"("error in (no error)"=w47, "AO Ref In"=w48) -> ()  [unwired: 9 in, 1 out]
      n145 = call <vilib>:"Close.vi"("PWM Ref In"=w53) -> ()  [unwired: 10 in, 1 out]
      n146 = call <vilib>:"Close.vi"("error in (no error)"=w83, "DIO Ref In"=w84) -> ()  [unwired: 9 in, 1 out]
      n147 = call <vilib>:"Close.vi"("error in (no error)"=w66, "AO Ref In"=w67) -> ()  [unwired: 9 in, 1 out]
      n148 = call <vilib>:"Close.vi"("error in (no error)"=w73, "DIO Ref In"=w74) -> ()  [unwired: 9 in, 1 out]
      n149 = call <vilib>:"Close.vi"("error in (no error)"=w78, "PWM Ref In"=w79) -> ()  [unwired: 9 in, 1 out]
      n150 = TCP Close Connection(connection ID=w64, error in (no error)=w63) -> ()  [unwired: 1 in, 2 out]
      n151 = TCP Close Connection(connection ID=w58, error in (no error)=w59) -> ()  [unwired: 1 in, 2 out]
    }
  }
  n152 = flat-sequence {
    frame #0 {
      n153 = local write "manual speed"(0.0 ("manual speed")) -> ()
      n154 = local write "Manual Steering torque"(0.0 ("con_vs")) -> ()
      n155 = local write "Steering torque input"(TRUE ("Steering torque input")) -> ()
      n156 = local write "Velocity input"(FALSE ("Velocity input")) -> ()
      n157 = call "car_spec.vi"("Car_name"="Prius") -> ()  [unwired: 5 in, 6 out]
      "lane both" <- FALSE ("lane both")
    }
    frame #1 {
      n158 = while {
        stop <- FALSE stop-if-true
        n159 = flat-sequence {
          frame #0 {
            n160 = Wait Until Next ms Multiple(millisecond multiple=u32 10) -> ()  [unwired: 1 out]
          }
          frame #1 {
            n161 = global read "rio_Global.vi" "LCM PC"() -> (w353:T5)
            n162 = call "LCM_read.vi"("LCM"=w353) -> ("data"=w351:string, "ID"=w352:string)  [unwired: 7 in, 2 out]
            n163 = case shown="\"CON_INPUT_T\"" w352 {
              tunnel: w351 -> [_ w354]
              frame "False", Default {
              }
              frame "CON_INPUT_T" {
                n164 = global read "rio_Global.vi" "CON_INPUT_T"() -> (w356:T22)
                n165 = Unflatten From String(type=w356, binary string=w354, data includes array or string size? (T)=FALSE) -> (value=w355:T22, error out=w357:errorcluster)  [unwired: 2 in, 1 out]
                n166 = case shown="No Error" w357 {
                  tunnel: w355 -> [w361 _]
                  frame No Error {
                    n167 = Unbundle By Name(w361) -> ("ref_vel"=w360:dbl, "ref_steer"=w359:dbl)
                    n168 = global write "rio_Global.vi" "Ref_str_ang"(w359) -> ()
                    n169 = global write "rio_Global.vi" "Ref_VS"(w360) -> ()
                  }
                  frame Error {
                  }
                }
              }
            }
          }
          frame #2 {
            w382 = 2 ("index")
            w384 = 2 ("index")
            n170 = global read "rio_Global.vi" "M_lane_right"() -> (w367:dbl[])
            n171 = global read "rio_Global.vi" "M_lane_left"() -> (w366:dbl[])
            n172 = Index Array(array=w366, index=w384) -> (element=w385:dbl)
            n173 = Index Array(array=w367, index=w382) -> (element=w383:dbl)
            n174 = Greater Or Equal?(x=w385, y=w384) -> (x >= y?=w373:bool)
            n175 = Greater Or Equal?(x=w383, y=w382) -> (x >= y?=w374:bool)
            n176 = local read "lane both"() -> (w371:bool)
            n177 = Or(x=w373, y=w374) -> (x .or. y?=w372:bool)
            n178 = global read "rio_Global.vi" "C_Right light"() -> (w363:bool)
            n179 = And(x=w373, y=w374) -> (x .and. y?=w370:bool)
            n180 = global read "rio_Global.vi" "C_Left light"() -> (w364:bool)
            n181 = global read "rio_Global.vi" "C_VS_CAN"() -> (w365:dbl)
            n182 = And(x=w372, y=w371) -> (x .and. y?=w369:bool)
            n183 = Or(x=w370, y=w369) -> (x .or. y?=w368:bool)
            n184 = Not Exclusive Or(1:w363, 2:w364) -> (0:w380:bool)
            n185 = Greater?(x=w365, y=0.0) -> (0:w376:bool)
            n186 = disable-structure shown="Enabled" {
              disable-tunnel: [w389 TRUE] -> w381
              disable-tunnel: w380 -> [w388 _]
              disable-tunnel: w376 -> [w387 _]
              disable-tunnel: w368 -> [w386 _]
              frame Enabled {
                n187 = Compound Arithmetic op=AND(w386, w387, w388) -> (w389:bool)
              }
              frame Disabled {
              }
            }
            n188 = case shown="True" w381 {
              tunnel: [w394 w401] -> w377
              tunnel: w366 -> [_ w399]
              tunnel: w367 -> [_ w398]
              frame False {
                n189 = local write "lane both"(FALSE ("lane both")) -> ()
                n190 = global write "rio_Global.vi" "M_lane_center"(dbl[] [] ("M_lane_center")) -> ()
                n191 = global read "rio_Global.vi" "steering torque"() -> (w391:dbl)
                n192 = Multiply(x="forgetting", y=w391) -> (x*y=w394:dbl)
              }
              frame True {
                n193 = flat-sequence {
                  tunnel: [w408] -> w400
                  tunnel: w399 -> [w407]
                  tunnel: w398 -> [w406]
                  tunnel: [w456] -> w404
                  tunnel: [w455] -> w403
                  tunnel: w400 -> [w449]
                  tunnel: [w450] -> w396
                  tunnel: w404 -> [w510]
                  tunnel: w403 -> [w509]
                  tunnel: [w497] -> w402
                  tunnel: [w500] -> w397
                  tunnel: w396 -> [w500]
                  tunnel: w402 -> [w533]
                  tunnel: [w534] -> w401
                  tunnel: w397 -> [w531]
                  frame #0 {
                    w414 = 2 ("index")
                    w412 = 2 ("index")
                    n194 = Index Array(array=w407, index=w412) -> (element=w411:dbl)
                    n195 = Index Array(array=w406, index=w414) -> (element=w413:dbl)
                    n196 = Greater Or Equal?(x=w411, y=w412) -> (x >= y?=w405:bool)
                    n197 = Greater Or Equal?(x=w413, y=w414) -> (x >= y?=w410:bool)
                    n198 = And(x=w405, y=w410) -> (x .and. y?=w409:bool)
                    n199 = case shown="True" w409 {
                      tunnel: w407 -> [w436 w440]
                      tunnel: w406 -> [w431 w444]
                      tunnel: [w428 w445] -> w408
                      tunnel: w405 -> [w430 _]
                      frame False {
                        w423 = 0.2 ("y")
                        w426 = 5 ("index")
                        w435 = 5 ("index")
                        n200 = global read "rio_Global.vi" "overall width"() -> (w415:dbl)
                        n201 = Index Array(array=w436, index=w435) -> (element=w433:dbl)
                        n202 = Index Array(array=w431, index=w426) -> (element=w425:dbl)
                        n203 = global read "rio_Global.vi" "lane width"() -> (w416:dbl)
                        n204 = Multiply(x=w415, y=w423) -> (x*y=w421:dbl)
                        n205 = Add(x=w421, y=w423) -> (x+y=w417:dbl)
                        n206 = Add(x=1.0 ("y"), y=w421) -> (x+y=w418:dbl)
                        n207 = Multiply(x=w416, y=0.5) -> (x*y=w420:dbl)
                        n208 = In Range and Coerce(upper limit=w418, x=w420, lower limit=w417) -> (coerced(x)=w419:dbl)  [unwired: 1 out]
                        n209 = Add(x=w433, y=w419) -> (x+y=w432:dbl)
                        n210 = Subtract(x=w425, y=w419) -> (x-y=w424:dbl)
                        n211 = Replace Array Subset(array=w436, new element=w432, index=w435) -> (w429:dbl[])
                        n212 = Replace Array Subset(array=w431, new element=w424, index=w426) -> (w427:dbl[])
                        n213 = Select(t=w429, s=w430, f=w427) -> (s? t:f=w428:dbl[])
                      }
                      frame True {
                        n214 = Add(x=w440, y=w444) -> (x+y=w447:dbl[])
                        n215 = Index Array(array=w440, index=5) -> (element=w438:dbl)
                        n216 = Index Array(array=w444, index=5) -> (element=w442:dbl)
                        n217 = local write "lane both"(TRUE ("lane both")) -> ()
                        n218 = Subtract(x=w442, y=w438) -> (x-y=w437:dbl)
                        n219 = global write "rio_Global.vi" "lane width"(w437) -> ()
                        n220 = Multiply(x=0.5, y=w447) -> (x*y=w445:dbl[])
                      }
                    }
                  }
                  frame #1 {
                    n221 = global write "rio_Global.vi" "M_lane_center"(w449) -> ()
                    n222 = global read "rio_Global.vi" "C_VS_CAN"() -> (w448:dbl)
                    n223 = Index Array(array=w449, index=10) -> (element=w452:dbl)
                    n224 = disable-structure shown="Enabled" {
                      disable-tunnel: w448 -> [w489 w490]
                      disable-tunnel: [w480 w494] -> w455
                      disable-tunnel: w452 -> [w474 _]
                      frame Disabled {
                        n225 = Subtract(x=w474, y=15.0) -> (x-y=w472:dbl)
                        n226 = Subtract(x=w489, y=15.0) -> (x-y=w483:dbl)
                        n227 = Max & Min(x=w472, y=0.0) -> (max(x,y)=w471:dbl)  [unwired: 1 out]
                        n228 = Max & Min(x=w483, y=0.0) -> (max(x,y)=w482:dbl)  [unwired: 1 out]
                        n229 = Multiply(x=w471, y=2.0) -> (x*y=w479:dbl)
                        n230 = Multiply(x=w482, y=2.0) -> (x*y=w486:dbl)
                        n231 = Round Toward -Infinity(1:w479) -> (0:w470:dbl)
                        n232 = Round Toward -Infinity(1:w486) -> (0:w485:dbl)
                        n233 = Increment(x=w470) -> (x+1=w469:dbl)
                        n234 = Increment(x=w485) -> (x+1=w477:dbl)
                        n235 = global read "rio_Global.vi" "x_view"() -> (w468:dbl[])
                        n236 = Max & Min(x=w469, y=w477) -> (min(x,y)=w476:dbl)  [unwired: 1 out]
                        n237 = Array Subset(array=w468, index=0, length=w476) -> (w480:dbl[])
                      }
                      frame Enabled {
                        n238 = Max & Min(x=15.0, y=w490) -> (max(x,y)=w493:dbl)  [unwired: 1 out]
                        n239 = Max & Min(x=50.0, y=w493) -> (min(x,y)=w492:dbl)  [unwired: 1 out]
                        n240 = Build Array(w492) -> (w494:dbl[])
                      }
                    }
                    n241 = Index Array(array=w449, index #1=5 ("index"), index #2=7 ("index"), index #3=6 ("index"), index #4=9 ("index"), index #5=5 ("index")) -> (element #1=w450:dbl, element #2=w466:dbl, element #3=w464:dbl, element #4=w462:dbl, element #5=w458:dbl)
                    n242 = Square(x=w455) -> (x^2=w454:dbl[])
                    n243 = Compound Arithmetic op=MULTIPLY(w454, w464) -> (w460:dbl[])
                    n244 = Compound Arithmetic op=MULTIPLY(w466, w455, w454) -> (w461:dbl[])
                    n245 = Compound Arithmetic op=MULTIPLY(w455, w462) -> (w459:dbl[])
                    n246 = Compound Arithmetic op=ADD(w461, w460, w459, w458) -> (w456:dbl[])
                  }
                  frame #2 {
                    n247 = for {
                      tunnel: [w516] -> w505 mode=indexing
                      tunnel: w510 -> [w520] mode=indexing
                      tunnel: w509 -> [w518] mode=indexing
                      tunnel: [1.0] -> w504 mode=indexing
                      n248 = Square(x=w520) -> (x^2=w523:dbl)
                      n249 = Square(x=w518) -> (x^2=w524:dbl)
                      n250 = Sign(1:w520) -> (0:w519:dbl)
                      n251 = Absolute Value(x=w520) -> (abs(x)=w522:dbl)
                      n252 = Multiply(x=w518, y=w519) -> (x*y=w517:dbl)
                      n253 = Greater Or Equal?(x=w522, y=w518) -> (x >= y?=w521:bool)
                      n254 = Add(x=w523, y=w524) -> (x+y=w525:dbl)
                      n255 = Divide(x=w525, y=w520) -> (x/y=w526:dbl)
                      n256 = Multiply(x=w526, y=0.5) -> (x*y=w528:dbl)
                      n257 = Select(t=w517, s=w521, f=w528) -> (s? t:f=w516:dbl)
                    }
                    n258 = Add Array Elements(numeric array=w504) -> (sum=w503:dbl)
                    n259 = Multiply(x=w505, y="gain(<1)") -> (x*y=w496:dbl[])
                    n260 = Add Array Elements(numeric array=w496) -> (sum=w507:dbl)
                    n261 = global read "rio_Global.vi" "wheel base"() -> (w499:dbl)
                    n262 = Divide(x=w507, y=w503) -> (x/y=w502:dbl)
                    n263 = Divide(x=w499, y=w502) -> (x/y=w501:dbl)
                    n264 = Inverse Tangent(1:w501) -> (0:w511:dbl)
                    n265 = Multiply(x=w511, y=180.0) -> (x*y=w513:dbl)
                    n266 = Divide(x=w513, y=3.141592653589793) -> (x/y=w508:dbl)
                    n267 = global read "rio_Global.vi" "ratio"() -> (w498:dbl)
                    n268 = Multiply(x=w498, y=w508) -> (x*y=w497:dbl)
                    "cmd steer" <- w497
                    n269 = global write "rio_Global.vi" "cmd steer"(w497) -> ()
                  }
                  frame #3 {
                    n270 = global read "rio_Global.vi" "C_mdps str_ang"() -> (w529:dbl)
                    n271 = Subtract(x=w533, y=w529) -> (x-y=w532:dbl)
                    n272 = disable-structure shown="Enabled" {
                      disable-tunnel: [w547 w585] -> w534
                      disable-tunnel: w533 -> [w545 _]
                      disable-tunnel: w532 -> [w539 w580]
                      disable-tunnel: w531 -> [w537 _]
                      disable-tunnel: "Kp" -> [w535 w586]
                      frame Disabled {
                        n273 = Square(x=w539) -> (x^2=w540:dbl)
                        n274 = Absolute Value(x=w539) -> (abs(x)=w538:dbl)
                        n275 = Multiply(x=w540, y=w539) -> (x*y=w542:dbl)
                        n276 = Greater Or Equal?(x=w538, y=1.0) -> (x >= y?=w543:bool)
                        n277 = Select(t=w542, s=w543, f=w539) -> (s? t:f=w541:dbl)
                        n278 = Multiply(x=w541, y=0.002) -> (x*y=w536:dbl)
                        n279 = Multiply(x=w535, y=w536) -> (x*y=w546:dbl)
                        n280 = disable-structure shown="Disabled" {
                          disable-tunnel: [w555 w574] -> w547
                          disable-tunnel: w546 -> [w549 w575]
                          disable-tunnel: w545 -> [_ w565]
                          disable-tunnel: w537 -> [_ w562]
                          frame Disabled {
                            n281 = Absolute Value(x=w549) -> (abs(x)=w554:dbl)
                            n282 = Greater?(x=w554, y="deadzone") -> (0:w553:bool)
                            n283 = Negate(x="visco") -> (-x=w557:dbl)
                            n284 = Select(t=w549, s=w553, f=0.0) -> (s? t:f=w550:dbl)
                            n285 = call "visco.vi"("min"=w557, "max"="visco", "input"=w550) -> ("output"=w555:dbl)  [unwired: 8 in]
                          }
                          frame Enabled {
                            n286 = Square(x=w565) -> (x^2=w566:dbl)
                            n287 = Multiply(x=w566, y=w565) -> (x*y=w564:dbl)
                            n288 = Multiply(x=w562, y="lane center") -> (x*y=w561:dbl)
                            n289 = Multiply(x=0.002 ("y"), y=w564) -> (x*y=w572:dbl)
                            n290 = In Range and Coerce(upper limit=0.2, x=w561, lower limit=-0.2) -> (coerced(x)=w558:dbl)  [unwired: 1 out]
                            n291 = Multiply(x="Kf", y=w572) -> (x*y=w568:dbl)
                            n292 = In Range and Coerce(upper limit=0.35, x=w568, lower limit=-0.35) -> (coerced(x)=w567:dbl)  [unwired: 1 out]
                            n293 = Compound Arithmetic op=ADD(w558, w567, w575) -> (w574:dbl)
                          }
                        }
                      }
                      frame Enabled {
                        n294 = Divide(x=w580, y=3.0) -> (x/y=w578:dbl)
                        n295 = Compound Arithmetic op=MULTIPLY(w578, w578, w578) -> (w577:dbl)
                        n296 = local read "rate limit"() -> (w583:dbl)
                        n297 = Multiply(x=w577, y=0.0001) -> (x*y=w587:dbl)
                        n298 = global read "rio_Global.vi" "steering torque"() -> (w576:dbl)
                        n299 = Multiply(x=w586, y=w587) -> (x*y=w584:dbl)
                        n300 = Negate(x=w583) -> (-x=w582:dbl)
                        n301 = In Range and Coerce(upper limit=w583, x=w584, lower limit=w582) -> (coerced(x)=w581:dbl)  [unwired: 1 out]
                        n302 = Add(x=w581, y=w576) -> (x+y=w585:dbl)
                        "Numeric" <- w580
                      }
                    }
                  }
                }
              }
            }
            n303 = In Range and Coerce(upper limit=0.4, x=w377, lower limit=-0.4) -> (coerced(x)=w362:dbl)  [unwired: 1 out]
            n304 = global write "rio_Global.vi" "Ref_str_torque"(w362) -> ()
          }
          frame #3 {
            w598 = 3.6  # m/2tokm/h
            w600 = 5.0  # 0.5g
            n305 = global read "rio_Global.vi" "M_headway"() -> (w595:dbl)
            n306 = global read "rio_Global.vi" "C_APV"() -> (→"APV":dbl)
            n307 = global read "rio_Global.vi" "Ref_VS"() -> (w589:dbl)
            n308 = Select(t=w589, s="Velocity input", f="manual speed") -> (s? t:f=w604:dbl)
            n309 = Multiply(x=w600, y=w595) -> (x*y=w599:dbl)
            n310 = disable-structure shown="Enabled" {
              disable-tunnel: w604 -> [w613 w644]
              disable-tunnel: [w612 w641] -> w603
              disable-tunnel: [_ w640] -> w590
              frame Disabled {
                n311 = flat-sequence {
                  tunnel: w613 -> [w638]
                  tunnel: [w637] -> w612
                  frame #0 {
                    w620 = dbl[] [0.016, 0.025, 0.08]  # V_PID_gain
                    n312 = global read "rio_Global.vi" "C_VS_CAN"() -> (w614:dbl)
                    n313 = Subtract(x=w638, y=w614) -> (x-y=w639:dbl)
                    n314 = In Range and Coerce(upper limit=20.0, x=w639, lower limit=-999.0) -> (coerced(x)=w616:dbl)  [unwired: 1 out]
                    n315 = Absolute Value(x=w616) -> (abs(x)=w624:dbl)
                    n316 = feedback #1(w616) -> (w618:dbl)
                    n317 = feedback-in #1(w616) -> ()
                    n318 = Multiply(x=w616, y=0.01) -> (x*y=w634:dbl)
                    n319 = Subtract(x=w616, y=w618) -> (x-y=w617:dbl)
                    n320 = Greater?(x=w624, y=1.0) -> (0:w621:bool)
                    n321 = Select(t=w616, s=w621, f=0.0) -> (s? t:f=w631:dbl)
                    n322 = feedback #2(0.0) -> (w633:dbl)
                    n323 = Multiply(x=w633, y=0.95) -> (x*y=w627:dbl)
                    n324 = Add(x=w627, y=w634) -> (x+y=w628:dbl)
                    n325 = feedback-in #2(w628) -> ()
                    n326 = Divide(x=w617, y=0.01) -> (x/y=w615:dbl)
                    n327 = Build Array(w631, w628, w615) -> (w630:dbl[])
                    n328 = Multiply(x=w620, y=w630) -> (x*y=w629:dbl[])
                    n329 = Add Array Elements(numeric array=w629) -> (sum=w637:dbl)
                  }
                }
              }
              frame Enabled {
                n330 = global read "rio_Global.vi" "PWM GAS"() -> (w656:dbl)
                n331 = Subtract(x=w656, y=1000.0) -> (x-y=w653:dbl)
                n332 = global read "rio_Global.vi" "C_VS_CAN"() -> (w640:dbl)
                n333 = Multiply(x=w653, y=0.1) -> (x*y=w642:dbl)
                n334 = Subtract(x=w644, y=w640) -> (x-y=w643:dbl)
                n335 = feedback-in #3(w642) -> ()
                n336 = feedback #3(0.0) -> (w648:dbl)
                n337 = feedback #4(0.0) -> (w646:dbl)
                n338 = feedback-in #4(w640) -> ()
                n339 = Subtract(x=w642, y=w648) -> (x-y=w647:dbl)
                n340 = Equal?(x=w642, y=w648) -> (x = y?=w649:bool)
                n341 = Subtract(x=w640, y=w646) -> (x-y=w645:dbl)
                n342 = Equal?(x=w640, y=w646) -> (x = y?=w650:bool)
                n343 = case shown="False" w650 {
                  tunnel: w649 -> [_ w674]
                  tunnel: w647 -> [w670 _]
                  tunnel: w645 -> [w669 _]
                  tunnel: w643 -> [w668 w672]
                  tunnel: w642 -> [w667 w671]
                  tunnel: [w666 w673] -> w641
                  frame False {
                    n344 = Divide(x=w670, y=w669) -> (x/y=w661:dbl)
                    n345 = Absolute Value(x=w661) -> (abs(x)=w660:dbl)
                    n346 = In Range and Coerce(upper limit="upper limit", x=w660, lower limit=0.01) -> (coerced(x)=w657:dbl)  [unwired: 1 out]
                    n347 = Multiply(x=w668, y=w657) -> (x*y=w663:dbl)
                    n348 = In Range and Coerce(upper limit=25.0, x=w663, lower limit=-25.0) -> (coerced(x)=w662:dbl)  [unwired: 1 out]
                    n349 = Add(x=w667, y=w662) -> (x+y=w666:dbl)
                  }
                  frame True {
                    n350 = case shown="False" w674 {
                      tunnel: [w679 w684] -> w673
                      tunnel: w672 -> [w678 w683]
                      tunnel: w671 -> [w680 w681]
                      frame False {
                        n351 = In Range and Coerce(upper limit=5.0, x=w678, lower limit=-5.0) -> (coerced(x)=w677:dbl)  [unwired: 1 out]
                        n352 = Add(x=w680, y=w677) -> (x+y=w679:dbl)
                      }
                      frame True {
                        n353 = Equal To 0?(x=w683) -> (x = 0?=w682:bool)
                        n354 = case shown="False" w682 {
                          tunnel: w683 -> [w688 _]
                          tunnel: [w685 w689] -> w684
                          tunnel: w681 -> [_ w689]
                          frame False {
                            n355 = In Range and Coerce(upper limit=1.0, x=w688, lower limit=-1.0) -> (coerced(x)=w685:dbl)  [unwired: 1 out]
                          }
                          frame True {
                          }
                        }
                      }
                    }
                  }
                }
              }
            }
            "VS_CAN" <- w590
            n356 = Multiply(x=w598, y=w599) -> (x*y=→"recomammed Speed [km/h]":dbl)
            n357 = Not Equal To 0?(x=w604) -> (x != 0?=w601:bool)
            n358 = global read "rio_Global.vi" "C_MCP"() -> (w594:dbl)
            n359 = local read "T out"() -> (w606:i32)
            n360 = global read "rio_Global.vi" "Auto"() -> (w593:bool)
            "Auto" <- w593
            n361 = local read "T init"() -> (w605:i32)
            n362 = Greater Or Equal?(x=w605, y=w606) -> (x >= y?=w602:bool)
            n363 = Less?(x=w594, y=5.0) -> (x < y?=w608:bool)
            n364 = Compound Arithmetic op=AND(w602, w608, w593, w601) -> (w607:bool)
            n365 = case shown="False" w607 {
              tunnel: [1000.0 ("Numeric") w703] -> w592
              tunnel: w603 -> [_ w709]
              tunnel: w606 -> [w690 _]
              tunnel: [_ TRUE] -> w591
              frame False {
                n366 = local read "T init"() -> (w691:i32)
                n367 = Less Or Equal?(x=w691, y=w690) -> (x <= y?=w692:bool)
                n368 = case shown="True" w692 {
                  tunnel: w690 -> [_ w695]
                  frame False {
                    n369 = local write "T init"(1 ("T init")) -> ()
                  }
                  frame True {
                    n370 = local read "T init"() -> (w698:i32)
                    n371 = Increment(x=w698) -> (x+1=w697:i32)
                    n372 = Max & Min(x=w697, y=w695) -> (min(x,y)=w696:i32)  [unwired: 1 out]
                    n373 = local write "T init"(w696) -> ()
                  }
                }
              }
              frame True {
                w702 = 1000.0 ("x")
                n374 = disable-structure shown="Enabled" {
                  disable-tunnel: [w715 1000.0 ("PWM GAS")] -> w704
                  frame Disabled {
                    n375 = global read "rio_Global.vi" "PWM GAS"() -> (w715:dbl)
                  }
                  frame Enabled {
                  }
                }
                n376 = Multiply(x=10.0, y=w709) -> (x*y=w707:dbl)
                n377 = Add(x=w707, y=w704) -> (x+y=w706:dbl)
                n378 = In Range and Coerce(upper limit=1700.0, x=w706, lower limit=w702) -> (coerced(x)=w703:dbl)  [unwired: 1 out]
                n379 = Subtract(x=w703, y=w702) -> (x-y=w701:dbl)
                n380 = Multiply(x=w701, y=0.1) -> (x*y=w699:dbl)
                n381 = To Long Integer(number=w699) -> (32bit integer=w711:i32)
                n382 = Add(x=w711, y=20) -> (x+y=w713:i32)
                "T out" <- w713
                n383 = Increment(x=w713) -> (x+1=→"T init":i32)
              }
            }
            "PWM GAS" <- w592
            n384 = global write "rio_Global.vi" "Solenoid"(w591) -> ()
            n385 = global write "rio_Global.vi" "PWM GAS"(w592) -> ()
          }
          frame #4 {
            n386 = global read "rio_Global.vi" "C_mdps str_ang"() -> (→"mdps str_ang":dbl)
            n387 = global read "rio_Global.vi" "steering torque"() -> (w721:dbl)
            n388 = global read "rio_Global.vi" "C_mdps torque volt"() -> (w718:dbl)
            n389 = global read "rio_Global.vi" "Ref_str_ang"() -> (w717:dbl)
            n390 = Add(x="rate limit", y=w721) -> (x+y=w728:dbl)
            n391 = Subtract(x=w721, y="rate limit") -> (x-y=w727:dbl)
            n392 = Select(t=w717, s="Steering torque input", f="Manual Steering torque") -> (s? t:f=w723:dbl)
            n393 = In Range and Coerce(upper limit=w728, x=w723, lower limit=w727) -> (coerced(x)=w724:dbl)  [unwired: 1 out]
            n394 = Negate(x=w718) -> (-x=w726:dbl)
            "mdps torque volt" <- w726
            n395 = global read "rio_Global.vi" "Auto"() -> (w719:bool)
            n396 = Merge Signals(w723, w726) -> (→"Waveform Chart":dynamicdata)
            n397 = Select(t=w724, s=w719, f=0.0) -> (s? t:f=w720:dbl)
            n398 = global write "rio_Global.vi" "steering torque"(w720) -> ()
          }
          frame #5 {
            n399 = global read "rio_Global.vi" "C_gear selector disp"() -> (w733:u8)
            "Ring" <- w733
            n400 = global read "rio_Global.vi" "C_gear selector disp"() -> (w734:u8)
            n401 = Decimal String To Number(string="gear input", default (0L)=u8 0) -> (number=w735:u8)  [unwired: 1 in, 1 out]
            n402 = Not Equal?(x=w735, y=w734) -> (x != y?=w741:bool)
            n403 = Number To Decimal String(number=w733) -> (decimal integer string=→"current gear":string)  [unwired: 1 in]
            n404 = Select(t=w735, s=w741, f=u8 0) -> (s? t:f=w739:u8)
            n405 = case shown="3" w739 {
              frame 1 {
                n406 = global write "rio_Global.vi" "gear command set"(dbl[] [2.0, -2.0]) -> ()
              }
              frame 3 {
                n407 = global write "rio_Global.vi" "gear command set"(dbl[] [2.0, 2.0]) -> ()
              }
              frame 0, Default {
                n408 = global write "rio_Global.vi" "gear command set"(dbl[] [0.0, 0.0] ("gear command set")) -> ()
              }
            }
          }
        }
      }
    }
  }
  n409 = flat-sequence {
    tunnel: [w745] -> w1
    tunnel: w1 -> [w752]
    frame #0 {
      n410 = for {
        N: 257 -> [_]
        tunnel: [w751] -> w749 mode=indexing
        i -> [w751]
      }
      n411 = Multiply(x=w749, y=0.5) -> (x*y=w745:dbl[])
      n412 = Array Subset(array=w745, index=30) -> (w746:dbl[])  [unwired: 1 in]
      n413 = global write "rio_Global.vi" "x_view"(w746) -> ()
    }
    frame #1 {
      n414 = while {
        tunnel: w752 -> [w753]
        stop <- FALSE stop-if-true
        n415 = flat-sequence {
          tunnel: [w756] -> w754
          tunnel: w753 -> [w756]
          tunnel: w754 -> [w758]
          frame #0 {
            n416 = Wait Until Next ms Multiple(millisecond multiple=u32 33) -> ()  [unwired: 1 out]
          }
          frame #1 {
            n417 = call "mobileye_disp.vi"("x_view"=w758) -> ("XY Graph"=→"XY Graph":cluster{"Y":dbl[], "Y":dbl[]}[])  [unwired: 10 in]
          }
        }
      }
    }
  }
  n418 = disable-structure shown="Enabled" {
    frame Enabled {
      n419 = flat-sequence {
        tunnel: [dbl[] [0.0, 0.0, 0.0, 0.0, 0.0] ("pos(i)")] -> w760
        tunnel: w760 -> [w770]
        frame #0 {
          w763 = FALSE ("get heading")
          w764 = u64 1
          w761 = 0.0 ("dh_hat")
          w767 = 4 ("map")
          n420 = local write "GPS init"(w763) -> ()
          n421 = call "getecefdcmref.vi"("map"=w767) -> ("XYZ"=→"ecef ref":dbl[])  [unwired: 10 in, 4 out]
          "map" <- w767
          "vgain" <- 1.0 ("initH")
          "vcount" <- w764
          "hbias" <- w761
          "hcount" <- w764
          "get heading" <- w763
          "get position" <- w763
          "heading error" <- w761
          "h_gps" <- w761
          "rt" <- w761
          "pos error" <- w761
          "POS init" <- TRUE ("POS init")
        }
        frame #1 {
          n422 = flat-sequence {
            tunnel: [w1227] -> w769
            tunnel: w769 -> [w1235]
            frame #0 {
              n423 = while {
                shift-right: [w1233] -> w1229
                shift-left: refnum<visa-resource-name> "ASRL3::INSTR" ("VISA resource name") -> [w1234]
                stop <- w1232 continue-if-true
                n424 = VISA Open(VISA resource name=w1234) -> (VISA resource name=w1233:refnum<visa-resource-name>, error out=w1232:errorcluster)  [unwired: 4 in]
              }
              n425 = VISA Clear(VISA resource name=w1229) -> (VISA resource name out=w1231:refnum<visa-resource-name>)  [unwired: 1 in, 1 out]
              n426 = property class="Instr"(reference=w1231, "General Settings:Timeout Value"=u32 10) -> (reference out=w1227:refnum<visa-resource-name>)  [unwired: 1 in, 1 out]
            }
            frame #1 {
              n427 = while {
                tunnel: w1235 -> [w1236]
                stop <- FALSE stop-if-true
                n428 = flat-sequence {
                  tunnel: w1236 -> [w1238]
                  frame #0 {
                    n429 = VISA Read(VISA resource name=w1238, byte count=u32 100) -> (read buffer=w1239:string)  [unwired: 1 in, 3 out]
                    n430 = case shown="Default" w1239 {
                      selector: w1239 -> [_ w1241]
                      frame "" {
                      }
                      frame Default {
                        n431 = local read "ecef ref"() -> (w1242:dbl[])
                        n432 = call "nmea.vi"("ecef ref"=w1242, "NMEA"=w1241) -> ("output"=w1244:dbl[], "type"=w1243:u32)  [unwired: 8 in]
                        n433 = case shown="2" w1243 {
                          tunnel: w1244 -> [_ w1245 w1280]
                          frame 0, Default {
                          }
                          frame 1 {
                            n434 = disable-structure shown="Enabled" {
                              disable-tunnel: w1245 -> [w1247 _]
                              frame Enabled {
                                n435 = Index Array(array=w1247, index=1) -> (element=w1249:dbl)
                                n436 = Not Equal To 0?(x=w1249) -> (x != 0?=w1246:bool)
                                n437 = case shown="True" w1246 {
                                tunnel: w1247 -> [_ w1269]
                                frame False {
                                }
                                frame True {
                                n438 = Get Date/Time In Seconds() -> (seconds since 1Jan1904=w1254:timestamp)
                                n439 = To Double Precision Float(number=w1254) -> (double precision float=w1253:dbl)
                                n440 = global read "rio_Global.vi" "LCM_GGA_T"() -> (w1278:T23)
                                n441 = Array To Cluster(array=w1269) -> (cluster=w1277:T24)
                                n442 = Unbundle By Name(w1278) -> ("hash"=w1274:i64)
                                n443 = Multiply(x=w1253, y=1000000.0) -> (x*y=w1251:dbl)
                                n444 = Unbundle(w1277) -> ("output[0]"=w1279:dbl, "output[2]"=w1268:dbl, "output[3]"=w1267:dbl, "output[4]"=w1266:dbl, "output[6]"=w1265:dbl, "output[7]"=w1263:dbl, "output[8]"=w1261:dbl, "output[9]"=w1259:dbl, "output[12]"=w1258:dbl, "output[13]"=w1257:dbl, "output[14]"=w1256:dbl)  [unwired: 4 out]
                                n445 = To Quad Integer(1:w1251) -> (0:w1250:i64)
                                n446 = To Long Integer(number=w1265) -> (32bit integer=w1264:i32)
                                n447 = To Long Integer(number=w1263) -> (32bit integer=w1262:i32)
                                n448 = To Long Integer(number=w1261) -> (32bit integer=w1260:i32)
                                n449 = call "hash.vi"("input"=w1274) -> ("output"=w1273:i64)  [unwired: 10 in]
                                n450 = local read "map"() -> (w1255:i32)
                                n451 = Bundle(cluster=w1278, "hash"=w1273, "sys time"=w1250, "time"=w1279, "x"=w1268, "y"=w1267, "h"=w1266, "numSV"=w1264, "postype"=w1262, "lag"=w1260, "hordev"=w1259, "lat"=w1258, "lon"=w1257, "hgt"=w1256, "map_idx"=w1255) -> (w1275:T23)
                                n452 = Flatten To String(anything=w1275, prepend array or string size? (T)=FALSE) -> (data string=w1271:string)  [unwired: 2 in, 2 out]
                                n453 = global read "rio_Global.vi" "LCM"() -> (w1270:T5)
                                n454 = call "LCM_send.vi"("DATA"=w1271, "ID"="GGA_1", "LCM"=w1270) -> ()  [unwired: 6 in, 3 out]
                                }
                                }
                              }
                              frame Disabled {
                              }
                            }
                            n455 = global write "rio_Global.vi" "gps_pos 1"(w1245) -> ()
                          }
                          frame 2 {
                            n456 = disable-structure shown="Enabled" {
                              disable-tunnel: w1280 -> [w1284 _]
                              frame Enabled {
                                n457 = Index Array(array=w1284, index=1) -> (element=w1283:dbl)
                                n458 = Not Equal To 0?(x=w1283) -> (x != 0?=w1281:bool)
                                n459 = case shown="True" w1281 {
                                tunnel: w1284 -> [_ w1303]
                                frame False {
                                }
                                frame True {
                                n460 = Get Date/Time In Seconds() -> (seconds since 1Jan1904=w1289:timestamp)
                                n461 = To Double Precision Float(number=w1289) -> (double precision float=w1288:dbl)
                                n462 = global read "rio_Global.vi" "LCM_RMC_T"() -> (w1304:T25)
                                n463 = Unbundle By Name(w1304) -> ("hash"=w1300:i64)
                                n464 = Multiply(x=w1288, y=1000000.0) -> (x*y=w1286:dbl)
                                n465 = Array To Cluster(array=w1303) -> (cluster=w1302:T26)
                                n466 = To Quad Integer(1:w1286) -> (0:w1285:i64)
                                n467 = call "hash.vi"("input"=w1300) -> ("output"=w1299:i64)  [unwired: 10 in]
                                n468 = Unbundle(w1302) -> ("output[0]"=w1294:dbl, "output[2]"=w1293:dbl, "output[4]"=w1292:dbl, "output[5]"=w1291:dbl, "output[6]"=w1290:dbl)  [unwired: 2 out]
                                n469 = Bundle(cluster=w1304, "hash"=w1299, "sys time"=w1285, "time"=w1294, "speed"=w1293, "heading"=w1292, "lat"=w1291, "lon"=w1290) -> (w1295:T25)
                                n470 = Flatten To String(anything=w1295, prepend array or string size? (T)=FALSE) -> (data string=w1297:string)  [unwired: 2 in, 2 out]
                                n471 = global read "rio_Global.vi" "LCM"() -> (w1296:T5)
                                n472 = call "LCM_send.vi"("DATA"=w1297, "ID"="RMC_1", "LCM"=w1296) -> ()  [unwired: 6 in, 3 out]
                                }
                                }
                              }
                              frame Disabled {
                              }
                            }
                            n473 = global write "rio_Global.vi" "gps_vel 1"(w1280) -> ()
                          }
                        }
                      }
                    }
                  }
                }
              }
            }
          }
          n474 = disable-structure shown="Enabled" {
            disable-tunnel: w770 -> [w771 _]
            frame Enabled {
              n475 = while {
                shift-right: [w772] -> _
                shift-left: w771 -> [w773]
                stop <- FALSE stop-if-true
                n476 = flat-sequence {
                  tunnel: [w784] -> w776
                  tunnel: w773 -> [w784]
                  tunnel: w776 -> [w787]
                  tunnel: [w786] -> w775
                  tunnel: [w786] -> w774
                  tunnel: [w1200] -> w772
                  tunnel: w775 -> [w1201]
                  tunnel: w774 -> [w1200]
                  frame #0 {
                    n477 = global read "rio_Global.vi" "C_ts"() -> (→"dt":dbl)
                    n478 = Wait Until Next ms Multiple(millisecond multiple=u32 10) -> (millisecond timer value=w782:u32)
                    n479 = feedback #5(w782) -> (w781:u32)
                    n480 = feedback-in #5(w782) -> ()
                    n481 = Subtract(x=w782, y=w781) -> (x-y=w780:u32)
                    n482 = To Long Integer(number=w780) -> (32bit integer=→"Pos_time 10":i32)
                  }
                  frame #1 {
                    n483 = flat-sequence {
                      tunnel: w787 -> [w794]
                      tunnel: [w794] -> w785
                      tunnel: [w917] -> w786
                      tunnel: w785 -> [w918]
                      frame #0 {
                        n484 = disable-structure shown="Enabled" {
                          disable-tunnel: [w814 w815] -> w789
                          disable-tunnel: [w795 w816] -> w788
                          frame Disabled {
                            n485 = global read "rio_Global.vi" "gps_pos 1"() -> (w811:dbl[])
                            n486 = global read "rio_Global.vi" "gps_pos 2"() -> (w798:dbl[])
                            n487 = Add(x=w811, y=w798) -> (x+y=w813:dbl[])
                            n488 = Index Array(array=w811, index #1=0 ("index")) -> (element #1=w810:dbl, element #2=w809:dbl)  [unwired: 1 in]
                            n489 = Index Array(array=w798, index #1=0 ("index")) -> (element #1=w799:dbl, element #2=w800:dbl)  [unwired: 1 in]
                            n490 = feedback #6(w810) -> (w808:dbl)
                            n491 = feedback-in #6(w810) -> ()
                            n492 = feedback #7(w799) -> (w801:dbl)
                            n493 = feedback-in #7(w799) -> ()
                            n494 = Not Equal?(x=w810, y=w808) -> (x != y?=w807:bool)
                            n495 = Not Equal?(x=w799, y=w801) -> (x != y?=w802:bool)
                            n496 = Not Equal To 0?(x=w809) -> (x != 0?=w806:bool)
                            n497 = Not Equal To 0?(x=w800) -> (x != 0?=w803:bool)
                            n498 = And(x=w807, y=w806) -> (x .and. y?=w796:bool)
                            n499 = And(x=w802, y=w803) -> (x .and. y?=w797:bool)
                            n500 = And(x=w796, y=w797) -> (x .and. y?=w814:bool)
                            n501 = Multiply(x=w813, y=0.5) -> (x*y=w795:dbl[])
                          }
                          frame Enabled {
                            n502 = global read "rio_Global.vi" "gps_pos 1"() -> (w816:dbl[])
                            n503 = Index Array(array=w816, index #1=0 ("index")) -> (element #1=w822:dbl, element #2=w821:dbl)  [unwired: 1 in]
                            n504 = feedback #8(w822) -> (w820:dbl)
                            n505 = feedback-in #8(w822) -> ()
                            n506 = Not Equal?(x=w822, y=w820) -> (x != y?=w819:bool)
                            n507 = Not Equal To 0?(x=w821) -> (x != 0?=w818:bool)
                            n508 = And(x=w819, y=w818) -> (x .and. y?=w815:bool)
                          }
                        }
                        "pos_gps" <- w788
                        n509 = disable-structure shown="Enabled" {
                          disable-tunnel: [w868 w899] -> w793
                          disable-tunnel: [w867 w878] -> w792
                          disable-tunnel: [w839 w889] -> w791
                          disable-tunnel: [w827 w884] -> w790
                          frame Disabled {
                            n510 = global read "rio_Global.vi" "gps_vel 1"() -> (w866:dbl[])
                            n511 = global read "rio_Global.vi" "gps_vel 2"() -> (w845:dbl[])
                            n512 = Index Array(array=w866, index #1=0 ("index"), index #2=1 ("index"), index #3=4 ("index"), index #4=2 ("index")) -> (element #1=w857:dbl, element #2=w862:dbl, element #3=w859:dbl, element #4=w831:dbl)
                            n513 = Index Array(array=w845, index #1=0 ("index"), index #2=1 ("index"), index #3=4 ("index"), index #4=2 ("index")) -> (element #1=w854:dbl, element #2=w849:dbl, element #3=w852:dbl, element #4=w830:dbl)
                            n514 = global read "rio_Global.vi" "C_VS_CAN"() -> (w824:dbl)
                            n515 = global read "rio_Global.vi" "C_VS_CAN"() -> (w871:dbl)
                            n516 = Add(x=w831, y=w830) -> (x+y=w829:dbl)
                            n517 = Not Equal To 0?(x=w849) -> (x != 0?=w850:bool)
                            n518 = call "angleconv.vi"("deg"=w859) -> ("rad"=w842:dbl)  [unwired: 9 in, 1 out]
                            n519 = call "angleconv.vi"("deg"=w852) -> ("rad"=w841:dbl)  [unwired: 9 in, 1 out]
                            n520 = feedback #9(0.0 ("Real Matrix Element")) -> (w856:dbl)
                            n521 = feedback-in #9(w857) -> ()
                            n522 = feedback #10(0.0 ("Real Matrix Element")) -> (w855:dbl)
                            n523 = feedback-in #10(w854) -> ()
                            n524 = Not Equal?(x=w857, y=w856) -> (x != y?=w863:bool)
                            n525 = Not Equal?(x=w854, y=w855) -> (x != y?=w848:bool)
                            n526 = Not Equal To 0?(x=w862) -> (x != 0?=w861:bool)
                            n527 = Greater Or Equal To 0?(x=w871) -> (x >= 0?=w872:bool)
                            n528 = Absolute Value(x=w824) -> (abs(x)=w823:dbl)
                            n529 = Multiply(x=w829, y=0.5) -> (x*y=w838:dbl)
                            n530 = call "headingweightsum.vi"("a"=0.5, "h1"=w841, "h2"=w842) -> ("a*h2+(1-a)*h1"=w870:dbl)  [unwired: 8 in]
                            n531 = And(x=w863, y=w861) -> (x .and. y?=w844:bool)
                            n532 = And(x=w848, y=w850) -> (x .and. y?=w843:bool)
                            n533 = Divide(x=w838, y=w823) -> (x/y=w839:dbl)
                            n534 = Select(t=0.0, s=w872, f=3.141592653589793) -> (s? t:f=w869:dbl)
                            n535 = Decrement(x=w839) -> (x-1=w835:dbl)
                            n536 = call "headingoperater.vi"("h1"=w869, "h2"=w870) -> ("h2-h1"=w868:dbl)  [unwired: 8 in, 1 out]
                            n537 = And(x=w844, y=w843) -> (x .and. y?=w867:bool)
                            n538 = Absolute Value(x=w835) -> (abs(x)=w836:dbl)
                            n539 = Greater?(x=w823, y=15.0) -> (0:w825:bool)
                            n540 = Less?(x=w836, y=0.05) -> (x < y?=w828:bool)
                            n541 = Compound Arithmetic op=AND(w825, w828, w867) -> (w827:bool)
                          }
                          frame Enabled {
                            n542 = global read "rio_Global.vi" "gps_vel 1"() -> (w898:dbl[])
                            n543 = global read "rio_Global.vi" "C_VS_CAN"() -> (w882:dbl)
                            n544 = global read "rio_Global.vi" "C_VS_CAN"() -> (w901:dbl)
                            n545 = Index Array(array=w898, index #1=0 ("index"), index #2=1 ("index"), index #3=4 ("index"), index #4=2 ("index")) -> (element #1=w877:dbl, element #2=w894:dbl, element #3=w891:dbl, element #4=w880:dbl)
                            n546 = Greater Or Equal To 0?(x=w901) -> (x >= 0?=w902:bool)
                            n547 = Absolute Value(x=w882) -> (abs(x)=w881:dbl)
                            n548 = feedback #11(w877) -> (w890:dbl)
                            n549 = feedback-in #11(w877) -> ()
                            n550 = Divide(x=w880, y=w881) -> (x/y=w889:dbl)
                            n551 = call "angleconv.vi"("deg"=w891) -> ("rad"=w879:dbl)  [unwired: 9 in, 1 out]
                            n552 = Select(t=0.0, s=w902, f=3.141592653589793) -> (s? t:f=w900:dbl)
                            n553 = Not Equal?(x=w877, y=w890) -> (x != y?=w895:bool)
                            n554 = Not Equal To 0?(x=w894) -> (x != 0?=w893:bool)
                            n555 = Decrement(x=w889) -> (x-1=w886:dbl)
                            n556 = call "headingoperater.vi"("h1"=w900, "h2"=w879) -> ("h2-h1"=w899:dbl)  [unwired: 8 in, 1 out]
                            n557 = And(x=w895, y=w893) -> (x .and. y?=w878:bool)
                            n558 = Absolute Value(x=w886) -> (abs(x)=w887:dbl)
                            n559 = Greater?(x=w881, y=15.0) -> (0:w875:bool)
                            n560 = Less?(x=w887, y=0.05) -> (x < y?=w876:bool)
                            n561 = Compound Arithmetic op=AND(w878, w876, w875) -> (w884:bool)
                          }
                        }
                        n562 = local write "get position"(w789) -> ()
                        n563 = local write "h_gps"(w793) -> ()
                        n564 = case shown="True" w790 {
                          tunnel: w791 -> [_ w912]
                          frame False {
                          }
                          frame True {
                            w906 = u64 18446744073709551615
                            n565 = local read "vcount"() -> (w909:u64)
                            n566 = local read "vgain"() -> (w914:dbl)
                            n567 = Increment(x=w909) -> (x+1=w908:u64)
                            n568 = Not Equal?(x=w909, y=w906) -> (x != y?=w907:bool)
                            n569 = Multiply(x=w914, y=w909) -> (x*y=w913:dbl)
                            n570 = Add(x=w912, y=w913) -> (x+y=w911:dbl)
                            n571 = Select(t=w908, s=w907, f=w906) -> (s? t:f=w905:u64)
                            n572 = Divide(x=w911, y=w905) -> (x/y=w910:dbl)
                            n573 = local write "vcount"(w905) -> ()
                            n574 = local write "vgain"(w910) -> ()
                          }
                        }
                        n575 = local write "get heading"(w792) -> ()
                      }
                      frame #1 {
                        n576 = local read "dt"() -> (w916:dbl)
                        n577 = Greater Than 0?(x=w916) -> (x > 0?=w915:bool)
                        n578 = case shown="True" w915 {
                          tunnel: w918 -> [w919 w922]
                          tunnel: [w919 w921] -> w917
                          frame False {
                          }
                          frame True {
                            n579 = flat-sequence {
                              tunnel: w922 -> [w956]
                              tunnel: [w934] -> w920
                              tunnel: [w984] -> w921
                              tunnel: w920 -> [w983]
                              frame #0 {
                                n580 = global read "rio_Global.vi" "C_VS_CAN"() -> (w924:dbl)
                                n581 = Equal To 0?(x=w924) -> (x = 0?=w926:bool)
                                n582 = case shown="True" w926 {
                                tunnel: [w958 _] -> w925
                                frame False {
                                n583 = global read "rio_Global.vi" "C_yaw_rate"() -> (w957:dbl)
                                n584 = local read "hbias"() -> (w961:dbl)
                                n585 = Subtract(x=w957, y=w961) -> (x-y=w959:dbl)
                                n586 = Negate(x=w959) -> (-x=w960:dbl)
                                n587 = call "angleconv.vi"("deg"=w960) -> ("rad"=w958:dbl)  [unwired: 9 in, 1 out]
                                }
                                frame True {
                                w965 = u64 18446744073709551615
                                n588 = local read "hcount"() -> (w968:u64)
                                n589 = local read "hbias"() -> (w971:dbl)
                                n590 = Increment(x=w968) -> (x+1=w967:u64)
                                n591 = global read "rio_Global.vi" "C_yaw_rate"() -> (w962:dbl)
                                n592 = Not Equal?(x=w968, y=w965) -> (x != y?=w966:bool)
                                n593 = Multiply(x=w971, y=w968) -> (x*y=w970:dbl)
                                n594 = Add(x=w962, y=w970) -> (x+y=w969:dbl)
                                n595 = Select(t=w967, s=w966, f=w965) -> (s? t:f=w964:u64)
                                n596 = local write "hcount"(w964) -> ()
                                n597 = Divide(x=w969, y=w964) -> (x/y=w963:dbl)
                                n598 = local write "hbias"(w963) -> ()
                                }
                                }
                                n599 = global read "rio_Global.vi" "C_VS_CAN"() -> (w923:dbl)
                                n600 = local read "vgain"() -> (w929:dbl)
                                n601 = Multiply(x=w923, y=w929) -> (x*y=w928:dbl)
                                n602 = Divide(x=w928, y=3.6) -> (x/y=w927:dbl)
                                n603 = Index Array(array=w956, index #1=0 ("index"), index #2=3 ("index"), index #3=1 ("index"), index #4=3 ("index")) -> (element #1=w950:dbl, element #2=w948:dbl, element #3=w944:dbl, element #4=w939:dbl)
                                n604 = local read "dt"() -> (w953:dbl)
                                n605 = local read "dt"() -> (w937:dbl)
                                n606 = Multiply(x=w927, y=w953) -> (x*y=w949:dbl)
                                n607 = Multiply(x=w937, y=w925) -> (x*y=w930:dbl)
                                n608 = Cosine(x=w948) -> (cos(x)=w954:dbl)
                                n609 = Sine(x=w948) -> (sin(x)=w947:dbl)
                                n610 = Multiply(x=w954, y=w949) -> (x*y=w951:dbl)
                                n611 = Multiply(x=w949, y=w947) -> (x*y=w946:dbl)
                                n612 = local write "rt"(w930) -> ()
                                n613 = Add(x=w950, y=w951) -> (x+y=w943:dbl)
                                n614 = Add(x=w946, y=w944) -> (x+y=w942:dbl)
                                n615 = call "headingoperater.vi"("h1"=w930, "h2"=w939) -> ("h2+h1"=w938:dbl)  [unwired: 8 in, 1 out]
                                n616 = Build Array(w943, w942, w927, w938, w925) -> (w934:dbl[])
                                n617 = Index Array(array=w934, index=3) -> (element=w933:dbl)
                                n618 = local read "h_gps"() -> (w932:dbl)
                                n619 = call "headingoperater.vi"("h1"=w933, "h2"=w932) -> ("h2-h1"=w936:dbl)  [unwired: 8 in, 1 out]
                                n620 = Absolute Value(x=w936) -> (abs(x)=w931:dbl)
                                n621 = local write "heading error"(w931) -> ()
                              }
                              frame #1 {
                                n622 = local read "get heading"() -> (w991:bool)
                                n623 = local read "get position"() -> (w990:bool)
                                n624 = local read "POS init"() -> (w976:bool)
                                n625 = case shown="False" w976 {
                                tunnel: w991 -> [w994 w1001]
                                tunnel: w990 -> [w998 w1000]
                                tunnel: [w992 w999] -> w986
                                frame False {
                                n626 = local read "heading error"() -> (w995:dbl)
                                n627 = Less?(x=w995, y=0.05) -> (x < y?=w996:bool)
                                n628 = And(x=w994, y=w996) -> (x .and. y?=w993:bool)
                                n629 = Or(x=w993, y=w998) -> (x .or. y?=w992:bool)
                                }
                                frame True {
                                n630 = disable-structure shown="Enabled" {
                                disable-tunnel: w1001 -> [w1004 w1006]
                                disable-tunnel: w1000 -> [w1003 w1005]
                                disable-tunnel: [w1002 w1007] -> w999
                                frame Disabled {
                                n631 = And(x=w1004, y=w1003) -> (x .and. y?=w1002:bool)
                                }
                                frame Enabled {
                                n632 = Or(x=w1006, y=w1005) -> (x .or. y?=w1007:bool)
                                }
                                }
                                }
                                }
                                n633 = global read "rio_Global.vi" "C_VS_CAN"() -> (w989:dbl)
                                n634 = local read "heading error"() -> (w979:dbl)
                                n635 = Absolute Value(x=w989) -> (abs(x)=w988:dbl)
                                n636 = local read "POS init"() -> (w977:bool)
                                n637 = Greater?(x=w988, y=5.0) -> (0:w985:bool)
                                n638 = Less?(x=w979, y=1.0) -> (x < y?=w978:bool)
                                n639 = Or(x=w978, y=w977) -> (x .or. y?=w980:bool)
                                n640 = And(x=w986, y=w985) -> (x .and. y?=w981:bool)
                                n641 = And(x=w981, y=w980) -> (x .and. y?=w974:bool)
                                n642 = Select(t=FALSE, s="GPS init", f=w974) -> (s? t:f=w973:bool)
                                n643 = case shown="True" w973 {
                                tunnel: [w1011 w1040] -> w984
                                tunnel: w983 -> [w1012 w1043]
                                frame False {
                                n644 = global read "rio_Global.vi" "C_VS_CAN"() -> (w1015:dbl)
                                n645 = local read "POS init"() -> (w1014:bool)
                                n646 = Equal To 0?(x=w1015) -> (x = 0?=w1013:bool)
                                n647 = local read "GPS init"() -> (w1008:bool)
                                n648 = And(x=w1014, y=w1013) -> (x .and. y?=w1010:bool)
                                n649 = Or(x=w1010, y=w1008) -> (x .or. y?=w1009:bool)
                                n650 = case shown="True" w1009 {
                                tunnel: w1012 -> [w1016 w1017]
                                tunnel: [w1016 w1019] -> w1011
                                tunnel: w1008 -> [_ w1018]
                                frame False {
                                }
                                frame True {
                                n651 = case shown="False" w1018 {
                                tunnel: [w1030 w1039] -> w1019
                                tunnel: w1017 -> [w1025 w1033]
                                frame True {
                                n652 = Index Array(array=w1025, index #1=2 ("index")) -> (element #2=w1020:dbl, element #3=w1023:dbl)  [unwired: 2 in, 1 out]
                                n653 = local read "pos_gps"() -> (w1026:dbl[])
                                n654 = local write "GPS init"(FALSE ("GPS init")) -> ()
                                n655 = Index Array(array=w1026, index #1=2 ("index")) -> (element #1=w1028:dbl, element #2=w1027:dbl)  [unwired: 1 in]
                                n656 = local read "h_gps"() -> (w1021:dbl)
                                n657 = Build Array(w1028, w1027, w1020, w1021, w1023) -> (w1030:dbl[])
                                }
                                frame False {
                                w1032 = 0.0 ("element")
                                n658 = Index Array(array=w1033, index=3) -> (element=w1031:dbl)
                                n659 = local read "pos_gps"() -> (w1035:dbl[])
                                n660 = Index Array(array=w1035, index #1=2 ("index")) -> (element #1=w1037:dbl, element #2=w1036:dbl)  [unwired: 1 in]
                                n661 = Build Array(w1037, w1036, w1032, w1031, w1032) -> (w1039:dbl[])
                                }
                                }
                                }
                                }
                                }
                                frame True {
                                n662 = flat-sequence {
                                tunnel: w1043 -> [w1044]
                                tunnel: [w1044] -> w1042
                                tunnel: w1042 -> [w1085]
                                tunnel: [w1085] -> w1041
                                tunnel: w1041 -> [w1112]
                                tunnel: [w1116] -> w1040
                                frame #0 {
                                w1053 = 0.0 ("element")
                                w1057 = 0.0 ("element")
                                w1059 = 0.0 ("element")
                                w1061 = 0.0 ("element")
                                w1063 = 0.0 ("element")
                                n663 = Index Array(array=w1044, index #1=3 ("index"), index #2=2 ("index"), index #3=3 ("index"), index #4=2 ("index")) -> (element #1=w1073:dbl, element #2=w1075:dbl, element #3=w1078:dbl, element #4=w1067:dbl)
                                n664 = Negate(x=w1075) -> (-x=w1074:dbl)
                                n665 = Sine & Cosine(0:w1078) -> (1:w1070:dbl, 2:w1068:dbl)
                                n666 = Multiply(x=w1074, y=w1070) -> (x*y=w1071:dbl)
                                n667 = Multiply(x=w1068, y=w1067) -> (x*y=w1066:dbl)
                                n668 = Cosine(x=w1073) -> (cos(x)=w1072:dbl)
                                n669 = Build Array(w1063, w1063, w1072, w1071, 0.0 ("element")) -> (w1065:dbl[])
                                n670 = Build Array(w1061, w1061, w1070, w1066, 0.0 ("element")) -> (w1064:dbl[])
                                n671 = Build Array(w1059, w1059, w1059, w1059, w1059) -> (w1058:dbl[])
                                n672 = Build Array(w1057, w1057, w1057, w1057, 1.0 ("element")) -> (w1055:dbl[])
                                n673 = Build Array(w1053, w1053, w1053, w1053, w1053) -> (w1054:dbl[])
                                n674 = Build Array(w1065, w1064, w1058, w1055, w1054) -> (w1051:dbl[][])
                                n675 = call-poly <vilib>:"Array To Matrix.vi"("Real 2D Array"=w1051) -> ("Real Matrix"=w1049:T27)
                                n676 = global read "rio_Global.vi" "P"() -> (w1052:T27)
                                n677 = Transpose Matrix(1:w1049) -> (0:w1048:T27)
                                n678 = call-poly <vilib>:"Multiply.vi"("Real Matrix B"=w1052, "Real Matrix A"=w1049) -> ("A * B"=w1050:T27)
                                n679 = call-poly <vilib>:"Multiply.vi"("Real Matrix B"=w1048, "Real Matrix A"=w1050) -> ("A * B"=w1047:T27)
                                n680 = global read "rio_Global.vi" "Q"() -> (w1046:T27)
                                n681 = call-poly <vilib>:"Add.vi"("Real Matrix B"=w1046, "Real Matrix A"=w1047) -> ("A + B"=w1045:T27)
                                n682 = global write "rio_Global.vi" "Pp"(w1045) -> ()
                                }
                                frame #1 {
                                n683 = global read "rio_Global.vi" "Pp"() -> (w1110:T27)
                                n684 = global read "rio_Global.vi" "H"() -> (w1109:T27)
                                n685 = Array Subset(array=w1085, index=0, length=2) -> (w1092:dbl[])
                                n686 = local read "pos_gps"() -> (w1088:dbl[])
                                n687 = call-poly <vilib>:"Multiply.vi"("Real Matrix B"=w1110, "Real Matrix A"=w1109) -> ("A * B"=w1108:T27)
                                n688 = Transpose Matrix(1:w1109) -> (0:w1107:T27)
                                n689 = call-poly <vilib>:"Multiply.vi"("Real Matrix B"=w1107, "Real Matrix A"=w1108) -> ("A * B"=w1106:T27)
                                n690 = Array Subset(array=w1088, index=2, length=2) -> (w1091:dbl[])
                                n691 = Subtract(x=w1091, y=w1092) -> (x-y=w1093:dbl[])
                                n692 = global read "rio_Global.vi" "H"() -> (w1104:T27)
                                n693 = global read "rio_Global.vi" "R"() -> (w1105:T27)
                                n694 = local read "heading error"() -> (w1097:dbl)
                                n695 = global read "rio_Global.vi" "Pp"() -> (w1103:T27)
                                n696 = call-poly <vilib>:"Add.vi"("Real Matrix B"=w1105, "Real Matrix A"=w1106) -> ("A + B"=w1100:T27)
                                n697 = Square(x=w1093) -> (x^2=w1094:dbl[])
                                n698 = Transpose Matrix(1:w1104) -> (0:w1102:T27)
                                n699 = call-poly <vilib>:"Multiply.vi"("Real Matrix B"=w1102, "Real Matrix A"=w1103) -> ("A * B"=w1101:T27)
                                n700 = Add Array Elements(numeric array=w1094) -> (sum=w1095:dbl)
                                n701 = call-poly <vilib>:"Inverse Matrix.vi"("Input Matrix"=w1100) -> ("Inverse Matrix"=w1099:T27)  [unwired: 1 in, 1 out]
                                n702 = call-poly <vilib>:"Multiply.vi"("Real Matrix B"=w1099, "Real Matrix A"=w1101) -> ("A * B"=w1098:T27)
                                n703 = Square Root(x=w1095) -> (sqrt(x)=w1084:dbl)
                                n704 = global write "rio_Global.vi" "K"(w1098) -> ()
                                n705 = Less?(x=w1097, y=0.05) -> (x < y?=w1082:bool)
                                n706 = Less?(x=w1084, y=2.5) -> (x < y?=w1081:bool)
                                n707 = And(x=w1082, y=w1081) -> (x .and. y?=w1080:bool)
                                n708 = case shown="True" w1080 {
                                frame False {
                                }
                                frame True {
                                n709 = local write "POS init"(FALSE ("Kalman init")) -> ()
                                }
                                }
                                }
                                frame #2 {
                                n710 = disable-structure shown="Enabled" {
                                disable-tunnel: [w1128 w1129] -> w1115
                                frame Disabled {
                                n711 = local read "get heading"() -> (w1128:bool)
                                }
                                frame Enabled {
                                n712 = local read "heading error"() -> (w1132:dbl)
                                n713 = local read "POS init"() -> (w1130:bool)
                                n714 = Less?(x=w1132, y=0.1) -> (x < y?=w1131:bool)
                                n715 = Or(x=w1131, y=w1130) -> (x .or. y?=w1129:bool)
                                }
                                }
                                n716 = disable-structure shown="Enabled" {
                                disable-tunnel: [w1134 w1136] -> w1114
                                disable-tunnel: w1112 -> [_ w1145]
                                frame Disabled {
                                n717 = local read "get position"() -> (w1134:bool)
                                }
                                frame Enabled {
                                n718 = Array Subset(array=w1145, index=0, length=2) -> (w1143:dbl[])
                                n719 = local read "pos_gps"() -> (w1148:dbl[])
                                n720 = Array Subset(array=w1148, index=2, length=2) -> (w1144:dbl[])
                                n721 = disable-structure shown="Enabled" {
                                disable-tunnel: [w1151 TRUE ("Kalman init")] -> w1138
                                frame Disabled {
                                n722 = local read "POS init"() -> (w1151:bool)
                                }
                                frame Enabled {
                                }
                                }
                                n723 = Subtract(x=w1144, y=w1143) -> (x-y=w1142:dbl[])
                                n724 = Square(x=w1142) -> (x^2=w1141:dbl[])
                                n725 = Add Array Elements(numeric array=w1141) -> (sum=w1140:dbl)
                                n726 = Square Root(x=w1140) -> (sqrt(x)=w1135:dbl)
                                n727 = local write "pos error"(w1135) -> ()
                                n728 = Less?(x=w1135, y=3.0) -> (x < y?=w1137:bool)
                                n729 = Or(x=w1138, y=w1137) -> (x .or. y?=w1136:bool)
                                }
                                }
                                n730 = Index Array(array=w1112, index=3) -> (element=w1119:dbl)
                                n731 = global read "rio_Global.vi" "K"() -> (w1127:T27)
                                n732 = global read "rio_Global.vi" "H"() -> (w1126:T27)
                                n733 = global read "rio_Global.vi" "Pp"() -> (w1124:T27)
                                n734 = call-poly <vilib>:"Multiply.vi"("Real Matrix B"=w1126, "Real Matrix A"=w1127) -> ("A * B"=w1125:T27)
                                n735 = global read "rio_Global.vi" "Pp"() -> (w1122:T27)
                                n736 = call-poly <vilib>:"Multiply.vi"("Real Matrix B"=w1124, "Real Matrix A"=w1125) -> ("A * B"=w1123:T27)
                                n737 = call-poly <vilib>:"Subtract.vi"("Real Matrix B"=w1123, "Real Matrix A"=w1122) -> ("A - B"=w1121:T27)
                                n738 = global write "rio_Global.vi" "P"(w1121) -> ()
                                n739 = case shown="True" w1115 {
                                tunnel: w1119 -> [w1177 w1184]
                                tunnel: [w1177 w1179] -> w1113
                                frame False {
                                }
                                frame True {
                                n740 = global read "rio_Global.vi" "K"() -> (w1183:T27)
                                n741 = Index Array(array=w1183, index (row)=3, index (col)=2 ("disabled index (col)")) -> (element=w1180:dbl)
                                n742 = local read "h_gps"() -> (w1178:dbl)
                                n743 = call "headingweightsum2.vi"("a"=w1180, "h2"=w1178, "h1"=w1184) -> ("a*h2+(1-a)*h1"=w1179:dbl)  [unwired: 8 in]
                                }
                                }
                                n744 = case shown="True" w1114 {
                                tunnel: w1112 -> [w1153 w1165]
                                tunnel: [w1153 w1164] -> w1118
                                tunnel: w1113 -> [_ w1154]
                                frame False {
                                }
                                frame True {
                                n745 = disable-structure shown="Enabled" {
                                disable-tunnel: [w1175 w1176] -> w1155
                                disable-tunnel: w1154 -> [_ w1176]
                                frame Disabled {
                                n746 = local read "h_gps"() -> (w1175:dbl)
                                }
                                frame Enabled {
                                }
                                }
                                n747 = local read "pos_gps"() -> (w1159:dbl[])
                                n748 = call-poly <vilib>:"Array To Matrix.vi"("Real 1D Array"=w1165) -> ("Real Matrix (Column Vector)"=w1169:T27)
                                n749 = Array Subset(array=w1159, index=2, length=2) -> (w1160:dbl[])
                                n750 = Build Array (concatenate)(w1160, w1155) -> (w1156:dbl[])
                                n751 = global read "rio_Global.vi" "H"() -> (w1174:T27)
                                n752 = call-poly <vilib>:"Multiply.vi"("Real Matrix B"=w1169, "Real Matrix A"=w1174) -> ("A * B"=w1173:T27)
                                n753 = call-poly <vilib>:"Array To Matrix.vi"("Real 1D Array"=w1156) -> ("Real Matrix (Column Vector)"=w1172:T27)
                                n754 = call-poly <vilib>:"Subtract.vi"("Real Matrix B"=w1173, "Real Matrix A"=w1172) -> ("A - B"=w1170:T27)
                                n755 = global read "rio_Global.vi" "K"() -> (w1171:T27)
                                n756 = call-poly <vilib>:"Multiply.vi"("Real Matrix B"=w1170, "Real Matrix A"=w1171) -> ("A * B"=w1163:T27)
                                n757 = call-poly <vilib>:"Multiply.vi"("Real Matrix A"=w1163, "Real Scalar c"=0.25) -> ("c * A"=w1161:T27)
                                n758 = call-poly <vilib>:"Add.vi"("Real Matrix B"=w1169, "Real Matrix A"=w1161) -> ("A + B"=w1168:T27)
                                n759 = call-poly <vilib>:"Matrix To Array.vi"("Real Matrix"=w1168) -> ("Real 2D Array"=w1167:dbl[][])
                                n760 = Index Array(array=w1167, index (col)=0 ("disabled index (col)")) -> (element=w1164:dbl[])  [unwired: 1 in]
                                }
                                }
                                n761 = Replace Array Subset(array=w1118, new element=w1113, index=3) -> (w1116:dbl[])
                                }
                                }
                                }
                                }
                              }
                            }
                          }
                        }
                      }
                    }
                  }
                  frame #2 {
                    n762 = local read "h_gps"() -> (w1190:dbl)
                    n763 = local read "dt"() -> (w1187:dbl)
                    n764 = Index Array(array=w1201, index=3) -> (element=w1194:dbl)
                    n765 = Array Subset(array=w1201, index=0, length=2) -> (→"pos":dbl[])
                    n766 = Greater Than 0?(x=w1187) -> (x > 0?=w1186:bool)
                    n767 = call "angleconv.vi"("rad"=w1194) -> ("deg"=→"Heading":dbl)  [unwired: 9 in, 1 out]
                    n768 = Greater?(x=1.0, y=w1187) -> (0:w1189:bool)
                    n769 = call "headingoperater.vi"("h1"=0.0, "h2"=w1190) -> ("h2+h1"=w1191:dbl)  [unwired: 8 in, 1 out]
                    n770 = call "angleconv.vi"("rad"=w1191) -> ("deg"=→"H_GPS":dbl)  [unwired: 9 in, 1 out]
                    n771 = Compound Arithmetic op=AND(w1189, w1186) -> (w1185:bool)
                    n772 = case shown="True" w1185 {
                      tunnel: w1201 -> [_ w1202]
                      frame False {
                      }
                      frame True {
                        n773 = flat-sequence {
                          tunnel: w1202 -> [w1226]
                          frame #0 {
                            n774 = Get Date/Time In Seconds() -> (seconds since 1Jan1904=w1217:timestamp)
                            n775 = To Double Precision Float(number=w1217) -> (double precision float=w1211:dbl)
                            n776 = global read "rio_Global.vi" "LCM_POS_T"() -> (w1225:T28)
                            n777 = local read "POS init"() -> (w1207:bool)
                            n778 = Unbundle By Name(w1225) -> ("hash"=w1222:i64)
                            n779 = local read "dt"() -> (w1206:dbl)
                            n780 = Multiply(x=w1211, y=1000000.0) -> (x*y=w1209:dbl)
                            n781 = Array To Cluster(array=w1226) -> (cluster=w1224:T29)
                            n782 = Select(t=0.0, s=w1207, f=w1206) -> (s? t:f=w1204:dbl)
                            n783 = call "hash.vi"("input"=w1222) -> ("output"=w1221:i64)  [unwired: 10 in]
                            n784 = To Quad Integer(1:w1209) -> (0:w1208:i64)
                            n785 = Unbundle(w1224) -> ("Real 2D Array[0]"=w1216:dbl, "Real 2D Array[1]"=w1215:dbl, "Real 2D Array[2]"=w1214:dbl, "Real 2D Array[3]"=w1213:dbl, "Real 2D Array[4]"=w1212:dbl)
                            n786 = Bundle(cluster=w1225, "hash"=w1221, "sys time"=w1208, "dt"=w1204, "x"=w1216, "y"=w1215, "speed"=w1214, "heading"=w1213, "yaw_rate"=w1212) -> (w1203:T28)
                            n787 = Flatten To String(anything=w1203, prepend array or string size? (T)=FALSE) -> (data string=w1219:string)  [unwired: 2 in, 2 out]
                            n788 = global read "rio_Global.vi" "LCM"() -> (w1218:T5)
                            n789 = call "LCM_send.vi"("DATA"=w1219, "ID"="POS_T", "LCM"=w1218) -> ()  [unwired: 6 in, 3 out]
                          }
                        }
                      }
                    }
                  }
                }
              }
            }
            frame Disabled {
            }
          }
        }
      }
    }
    frame Disabled {
    }
  }
